vi "KM_fancytorque - ark - V2.vi.vi"() -> ()   [LabVIEW 2016]
uses:
  lorentzian.ctl
  circle corners.ctl
  <vilib>/event_ctls.llb/eventvkey.ctl
  peak -- parameters -- complex fit.ctl
  wavepacket.ctl
  filter method control.ctl
  cursor winow.ctl
  KM_SystemParameters.ctl
  parameters -- scan monitor control.ctl
  plot refs -- filter related.ctl
  cursor window action.ctl
  KM_ControlHFLIcommand.ctl
  KM_file -- read-write control.ctl
  filter - complex - four.vi
  linear interp iiii- complex - z-omega.vi
  peak -- PM find lorenzian - V3.vi
  tale of three indices.vi
  Q -- check range -- i -- real.vi
  filter -- window span logic.vi
  linear interp iiii- complex - z-omega - divide.vi
  linear interpolation iiii- complex.vi
  containing bix.vi
  <vilib>/Analysis/baseanly.llb/A x B.vi
  <vilib>/Analysis/baseanly.llb/Complex A x B.vi
  line -- complex.vi
  Q -- check range -- i -- integer.vi
  peak -- guess at omega -- dzdomega V2.vi
  command stack.vi
  tale of three indices -- check state.vi
  Q - not nan -- real.vi
  Q - not nan -- integer.vi
  peak -- z center from mult phase points.vi
  peak -- estimate for lorentzian.vi
  peak -- fake phase around center.vi
  peak -- get weights.vi
  peak -- four corner circle transformation logic.vi
  peak - fit phase around center - V2.vi
  array - generate range.vi
  circle center from three points.vi
  <vilib>/Utility/error.llb/Clear Errors.vi
  peak -- fit function -- minus arctan.vi
  <vilib>/Analysis/Matrix/Numeric/Conversions/Array To Matrix.vi
  <vilib>/Analysis/Matrix/Numeric/Conversions/Array To Matrix - RA2.vi
  <vilib>/Analysis/baseanly.llb/Inverse Matrix.vi
  <vilib>/Analysis/baseanly.llb/Real Inverse Matrix.vi
  <vilib>/gmath/NumericalOptimization/Nonlinear Curve Fit.vi
  <vilib>/gmath/NumericalOptimization/Nonlinear Curve Fit LM.vi
  KM_filter pipe - plot staff - more - V3.vi
panel:
  in  "Auto-update range":bool
  out "Plot: freq vs T":cluster{i32[], dbl[]}(graph)={[1, 2, 3, 4, 5, 6, 7, 8], [0.0, 0.0, 0.0, 0.0, 0.0, 0.0, 0.0, 0.0]}
  in  "scan monitor control":T1={"gamma acc. frac. - min "=0.3, "gamma acc frac.. - max"=3.0, "peak acc. fraction (af)"=5.0, "min peak acc. window (kHz)"=0.5, "use"=enum."fraction", "abs gamma min(kHz)"=0.005, "abs gamma max(kHz)"=5.0, "# points"=5, "gamma-factor (fa)"=12.0, "interpolate"=enum."line", "init"=TRUE, "Unique strike parameters"=TRUE, "max peak acc. window (kHz)"=10.0, "spacing factor"=1.5, "iterate #"=1, "overwrite ctl?"=FALSE, "write _m files?"=FALSE, "max slope (kHz/sweep)"=0.5, "funnel state"=enum."funnel open"}
  in  "Plot frequency shift":bool=TRUE
  in  "Tab : all plot":enum32{"Page 1"}(tab)
  in  "Save frequency scan":path=path "D:/data/TestFolder/1_test"
  in  "File name":string="lowT_turnonfield"
  in  "ZI HFLI System Parameters IN":T2={"IP Address"="DEV3523", "Start (Hz)"=44300.0, "Stop (Hz)"=44600.0, "Filter Order"=4, "Number of Points"=100, "Precision"=0, "Bandwidth (Hz)"=1.0, "Averaging"=1, "Log Sweep"=FALSE, "Demod"=0} {"Averaging" items=["1"=1, "2"=2, "4"=4, "16"=16, "32"=32, "64"=64]; "Bandwidth (Hz)" format="%#_p"; "Precision" items=["Low", "Med", "High"]; "Number of Points" min=2 max=66000; "Filter Order" items=["6, 1st"=1, "12, 2nd"=2, "18, 3rd"=3, "24, 4th"=4, "30, 5th"=5, "36, 6th"=6, "42, 7th"=7, "48, 8th"=8]; "Stop (Hz)" format="%_5p"; "Start (Hz)" format="%_5p"}
  in  "cursor bracket: All, data window":T3={"left"=43985.294117647056, "right "=45220.58823529412, "center"=44602.94117647059, "window"=1235.294117647063, "cursors"=[0, 1, 2], "relative"=2, "absolute"=2, "fixed vertical offset"=0.0, "vertical offset"=0.0, "skew"=0.0, "default window frac"=0.1, "kind"=enum."symmetric", "skew.left"=0.5, "skew.right"=0.5, "Plot ref"=refnum, "wing order"=enum."forw"}
  in  "Update system parameters":bool
  out "Plot: All":cluster{"all rows":dbl[], "all rows":dbl[]}[](graph)=[{"all rows"=[23781.086279042767, 37884.17530453629, 40730.30165309847, 41954.39033644089, 42636.5910965833, 43072.211915828164, 43374.97472640881, 43597.991322043665, 43769.395219758095, 43905.48114733492, 44016.33986360442, 44108.55436461339, 44186.60243501595, 44253.636077860036, 44311.93853542682, 44363.204457812426, 44408.71822460464, 44449.47114674833, 44486.24066879261, 44519.645208971815, 44550.18295396032, 44578.25983124116, 44604.21002541093, 44628.311259019785, 44650.7963336142, 44671.861957527966, 44691.67557714009, 44710.380719872854, 44728.10121457246, 44744.94455579366, 44761.00460863403, 44776.36380085277, 44791.094912919354, 44805.26255024563, 44818.924362350524, 44832.132059149895, 44844.93226360091, 44857.367231602824, 44869.47546368073, 44881.29222806208, 44892.85001093923, 44904.17890673009, 44915.30695880868, 44926.260459332385, 44937.06421533274, 44947.741787080384, 44958.31570381856, 44968.80766123682, 44979.238704490075, 44989.629400131525, 45000.0, 45010.370599868475, 45020.761295509925, 45031.19233876318, 45041.68429618144, 45052.258212919616, 45062.93578466726, 45073.739540667615, 45084.69304119132, 45095.82109326991, 45107.14998906077, 45118.70777193792, 45130.52453631927, 45142.632768397176, 45155.06773639909, 45167.867940850105, 45181.075637649476, 45194.73744975437, 45208.905087080646, 45223.63619914723, 45238.99539136597, 45255.05544420634, 45271.89878542754, 45289.619280127146, 45308.32442285991, 45328.138042472034, 45349.2036663858, 45371.688740980215, 45395.78997458907, 45421.74016875884, 45449.81704603968, 45480.354791028185, 45513.75933120739, 45550.52885325168, 45591.28177539536, 45636.79554218758, 45688.06146457318, 45746.363922139964, 45813.39756498405, 45891.44563538661, 45983.66013639558, 46094.51885266508, 46230.604780241905, 46402.008677956335, 46625.0252735912, 46927.788084171836, 47363.4089034167, 48045.60966355911, 49269.69834690153, 52115.82469546374], "all rows"=[1.507180397819642e-06, 3.0053428725600797e-06, 3.922075606503711e-06, 2.608239407945581e-06, 2.3153068786215975e-06, 2.1667159786404756e-06, 2.2480663150920602e-06, 2.1591637736680415e-06, 2.0406010131102796e-06, 1.8131660473052188e-06, 2.1641631962096037e-06, 1.6620790138843332e-06, 1.5483188951621796e-06, 1.0039220906155144e-06, 7.603105581707233e-07, -1.1257645296058376e-06, -4.067212706942762e-06, -9.665017348967127e-06, -2.7145929394177068e-05, -0.00015905859596686202, -0.00029765078861135373, -0.0005568586601063002, -7.503199898033523e-05, -2.4381034058832112e-05, -1.3732745859881554e-05, -9.162128154662954e-06, -5.7880575952868944e-06, -4.839254973019342e-06, -2.8674168905364767e-06, -2.511508572255624e-06, -1.9266065464564903e-06, -1.180561993162238e-06, -4.414876509949326e-07, -2.4995144900751636e-07, -2.306090385920931e-06, -3.32898094398004e-07, -2.3974866755640355e-07, 1.019240574116253e-07, 3.263816715050899e-08, 3.291312346419152e-07, 5.720671533295986e-07, 7.264601026105059e-07, 7.144153344906329e-07, 1.1467252526209203e-06, 1.3885442917260242e-07, 1.3569293842464745e-06, 4.986733167554071e-07, 9.04226425622522e-07, 8.405279148001506e-07, 9.635784680639955e-07, 9.025585600632723e-07, 9.53052489210983e-07, 1.064445276409997e-06, 9.414531610527688e-07, 1.1423376391833232e-06, 1.4404747200271967e-06, 1.1572303607929983e-06, 1.1489136925931929e-06, 1.1608344292377982e-06, 1.4063601012768658e-06, 1.1901130130630255e-06, 1.267385218460013e-06, 1.2134881757096428e-06, 1.3140538499450182e-06, 1.4380948660954965e-06, 1.4226762033262723e-06, 1.6676294224025657e-06, 1.4022384399448908e-06, 1.5332878307531674e-06, 1.3371392082792312e-06, 1.4812625899300352e-06, 1.5474023741165714e-06, 1.4765911352317293e-06, 1.5663869417997434e-06, 1.5191387016899292e-06, 1.5814603438757944e-06, 1.527339090381671e-06, 1.3993064074261812e-06, 1.3677070038810398e-06, 1.654406355267649e-06, 1.662451704615306e-06, 1.6023238691482394e-06, 1.643536308331802e-06, 1.715109028918168e-06, 1.7672201376857162e-06, 1.5898175608271295e-06, 1.6967535631888778e-06, 1.744979743776765e-06, 1.8004170427800995e-06, 1.6455601680772773e-06, 1.753509292922102e-06, 1.6387646743650107e-06, 1.8549056202586698e-06, 1.869763756168511e-06, 1.665830966011183e-06, 2.013303355058319e-06, 1.7103469358340893e-06, 1.7213577107899512e-06, 1.7921659681489454e-06, 1.4924510638264252e-06]}, {"all rows"=[23781.086279042767, 37884.17530453629, 40730.30165309847, 41954.39033644089, 42636.5910965833, 43072.211915828164, 43374.97472640881, 43597.991322043665, 43769.395219758095, 43905.48114733492, 44016.33986360442, 44108.55436461339, 44186.60243501595, 44253.636077860036, 44311.93853542682, 44363.204457812426, 44408.71822460464, 44449.47114674833, 44486.24066879261, 44519.645208971815, 44550.18295396032, 44578.25983124116, 44604.21002541093, 44628.311259019785, 44650.7963336142, 44671.861957527966, 44691.67557714009, 44710.380719872854, 44728.10121457246, 44744.94455579366, 44761.00460863403, 44776.36380085277, 44791.094912919354, 44805.26255024563, 44818.924362350524, 44832.132059149895, 44844.93226360091, 44857.367231602824, 44869.47546368073, 44881.29222806208, 44892.85001093923, 44904.17890673009, 44915.30695880868, 44926.260459332385, 44937.06421533274, 44947.741787080384, 44958.31570381856, 44968.80766123682, 44979.238704490075, 44989.629400131525, 45000.0, 45010.370599868475, 45020.761295509925, 45031.19233876318, 45041.68429618144, 45052.258212919616, 45062.93578466726, 45073.739540667615, 45084.69304119132, 45095.82109326991, 45107.14998906077, 45118.70777193792, 45130.52453631927, 45142.632768397176, 45155.06773639909, 45167.867940850105, 45181.075637649476, 45194.73744975437, 45208.905087080646, 45223.63619914723, 45238.99539136597, 45255.05544420634, 45271.89878542754, 45289.619280127146, 45308.32442285991, 45328.138042472034, 45349.2036663858, 45371.688740980215, 45395.78997458907, 45421.74016875884, 45449.81704603968, 45480.354791028185, 45513.75933120739, 45550.52885325168, 45591.28177539536, 45636.79554218758, 45688.06146457318, 45746.363922139964, 45813.39756498405, 45891.44563538661, 45983.66013639558, 46094.51885266508, 46230.604780241905, 46402.008677956335, 46625.0252735912, 46927.788084171836, 47363.4089034167, 48045.60966355911, 49269.69834690153, 52115.82469546374], "all rows"=[0.0007974563535224752, 0.0007996824585144777, 0.000801055863810559, 0.0008023709492684473, 0.0008043035904232198, 0.0008060221240327267, 0.0008079861588657607, 0.0008099138649989499, 0.0008137066342146559, 0.0008166912805273911, 0.0008200120682383414, 0.0008257743088013124, 0.0008309641548394156, 0.0008382418841201335, 0.0008461487511330439, 0.0008631010803868039, 0.0008811271703963326, 0.0009105163414004749, 0.0009569645659724035, 0.0010924084360759998, 0.0012057100706609103, 0.00029661926295813424, 0.0004983682064819104, 0.0006245092460519504, 0.0006642958975118122, 0.000688014953523849, 0.0007036528258253693, 0.0007157261277439108, 0.0007257539872476703, 0.0007312959968075897, 0.0007365652850056019, 0.000741597283698577, 0.0007446082694069566, 0.0007471174935341076, 0.0007503508253399753, 0.000751918924870222, 0.0007545834972275356, 0.0007563965356655345, 0.0007580560809787534, 0.0007597345506328334, 0.0007610640147972753, 0.0007620638516011741, 0.000763219604317757, 0.0007641855095685925, 0.0007646270699688182, 0.0007654766384662939, 0.0007665995562350204, 0.0007680602236370042, 0.0007685370065909853, 0.0007691156724573211, 0.0007697904764320084, 0.0007706588523945321, 0.0007710474382361046, 0.0007717486794004843, 0.0007720769775968043, 0.0007732272174720945, 0.0007736182720170691, 0.0007738807929827457, 0.0007742776555400716, 0.0007749620475055803, 0.0007754371345676591, 0.0007757086490079029, 0.0007762899207278298, 0.0007767543315421529, 0.0007771810290360273, 0.0007776882688728486, 0.0007779256746573937, 0.0007785274443675241, 0.0007789731848669883, 0.0007792025447058807, 0.000779593397699708, 0.000780229163960165, 0.0007805874509397673, 0.0007808925743319777, 0.0007811659957561538, 0.0007818848982870454, 0.0007824298317662446, 0.0007827009109037148, 0.0007832737586205113, 0.0007835664359312226, 0.0007840133213366123, 0.0007843433541846707, 0.0007848029218084065, 0.0007852955640946771, 0.000785941246910104, 0.0007862507459896485, 0.0007870285282892873, 0.000787403374663448, 0.0007878750037518486, 0.0007886287358713888, 0.0007892760304996889, 0.0007898803386809262, 0.0007905251121309694, 0.0007910664952091892, 0.0007919339457060896, 0.0007926132285289055, 0.0007933472670739158, 0.0007941997139364451, 0.0007955754573450963, 0.0007958472103074079]}]
  in  "Tab : everything":T4(tab)
  in  "Tab :  Fit controls":enum32{"complex plane", "complex plane 2"}(tab)
  in  "Plot: fragment - filter":cluster{dbl[], dbl[]}[](graph)=[{[44016.33986360442, 44108.55436461339, 44186.60243501595, 44253.636077860036, 44311.93853542682, 44363.204457812426, 44408.71822460464, 44449.47114674833, 44486.24066879261, 44519.645208971815, 44550.18295396032, 44578.25983124116, 44604.21002541093, 44628.311259019785, 44650.7963336142, 44671.861957527966, 44691.67557714009, 44710.380719872854, 44728.10121457246, 44744.94455579366, 44761.00460863403, 44776.36380085277, 44791.094912919354, 44805.26255024563, 44818.924362350524, 44832.132059149895, 44844.93226360091, 44857.367231602824, 44869.47546368073, 44881.29222806208, 44892.85001093923, 44904.17890673009, 44915.30695880868, 44926.260459332385, 44937.06421533274, 44947.741787080384, 44958.31570381856, 44968.80766123682, 44979.238704490075, 44989.629400131525, 45000.0, 45010.370599868475, 45020.761295509925, 45031.19233876318, 45041.68429618144, 45052.258212919616, 45062.93578466726, 45073.739540667615, 45084.69304119132, 45095.82109326991, 45107.14998906077, 45118.70777193792, 45130.52453631927, 45142.632768397176, 45155.06773639909, 45167.867940850105, 45181.075637649476, 45194.73744975437, 45208.905087080646], [3.2761277517625694e-05, 3.368662392853569e-05, 3.484817959260281e-05, 3.6103896069265395e-05, 3.780540521310197e-05, 4.01312562105535e-05, 4.1697056448412104e-05, 4.347218849800507e-05, 3.7907135227185645e-05, -5.6790609684878474e-05, -0.00016339047566297474, -0.0006374801230611212, -0.0001209044081063004, -4.0885266907126506e-05, -2.0811384583670646e-05, -1.0567441807905433e-05, -3.4639706146223517e-06, 4.146373059885665e-07, 4.783819783945139e-06, 6.487024951166878e-06, 8.345406755318776e-06, 1.0301866106267696e-05, 1.175628931342121e-05, 1.2556906642669138e-05, 1.1355840740066054e-05, 1.3653149534934326e-05, 1.4396450549924569e-05, 1.51720158795756e-05, 1.551153833224406e-05, 1.621032364967834e-05, 1.6771656102487094e-05, 1.716636559117661e-05, 1.7437922034212302e-05, 1.8093758491666083e-05, 1.7224831656009514e-05, 1.8613962643004104e-05, 1.8057064811010596e-05, 1.8808208984914108e-05, 1.886329540863593e-05, 1.9124404198964482e-05, 1.923061546287002e-05, 1.949237776515521e-05, 1.9695602411581522e-05, 1.9748210015891906e-05, 2.0023423103981333e-05, 2.0594351952506144e-05, 2.0415578199513682e-05, 2.0471849694701305e-05, 2.0580663842203036e-05, 2.0986422801630558e-05, 2.0893196741743764e-05, 2.1034651211649477e-05, 2.1124846709259075e-05, 2.133615640300294e-05, 2.1560983405099388e-05, 2.1670341368931204e-05, 2.1966004899596587e-05, 2.1856178916878592e-05, 2.2092467349835007e-05]}, {[44016.33986360442, 44108.55436461339, 44186.60243501595, 44253.636077860036, 44311.93853542682, 44363.204457812426, 44408.71822460464, 44449.47114674833, 44486.24066879261, 44519.645208971815, 44550.18295396032, 44578.25983124116, 44604.21002541093, 44628.311259019785, 44650.7963336142, 44671.861957527966, 44691.67557714009, 44710.380719872854, 44728.10121457246, 44744.94455579366, 44761.00460863403, 44776.36380085277, 44791.094912919354, 44805.26255024563, 44818.924362350524, 44832.132059149895, 44844.93226360091, 44857.367231602824, 44869.47546368073, 44881.29222806208, 44892.85001093923, 44904.17890673009, 44915.30695880868, 44926.260459332385, 44937.06421533274, 44947.741787080384, 44958.31570381856, 44968.80766123682, 44979.238704490075, 44989.629400131525, 45000.0, 45010.370599868475, 45020.761295509925, 45031.19233876318, 45041.68429618144, 45052.258212919616, 45062.93578466726, 45073.739540667615, 45084.69304119132, 45095.82109326991, 45107.14998906077, 45118.70777193792, 45130.52453631927, 45142.632768397176, 45155.06773639909, 45167.867940850105, 45181.075637649476, 45194.73744975437, 45208.905087080646], [4.0456808450971675e-05, 4.6166382765358476e-05, 5.1225852273429576e-05, 5.841507250197021e-05, 6.614053424687782e-05, 8.303814246526989e-05, 0.00010123540346869319, 0.00013110022718033595, 0.00018041604648722388, 0.0003440569052588822, 0.0004878676309891713, -0.00032997943510847485, -0.00025246106113384256, -0.00014257921935351738, -0.00010661530793636916, -8.473961821658563e-05, -7.040545973886184e-05, -5.893282942883901e-05, -4.969397906069325e-05, -4.440818367573857e-05, -3.944291172311682e-05, -3.47471838637017e-05, -3.200913365345908e-05, -2.9623362556086906e-05, -2.598473883380795e-05, -2.4948015024345428e-05, -2.238752166091039e-05, -2.071350043998997e-05, -1.9087580489515707e-05, -1.7532952688762136e-05, -1.6303563123755355e-05, -1.537205078526659e-05, -1.4248588940532444e-05, -1.3418081047746337e-05, -1.2742991914311553e-05, -1.2217836385869973e-05, -1.0918831921894665e-05, -9.602091623528738e-06, -9.124237073053972e-06, -8.593371908314502e-06, -7.924191065159315e-06, -7.094668945941207e-06, -6.7452307505540495e-06, -6.035231686449502e-06, -5.766174006007096e-06, -4.7240714488641515e-06, -4.275528285473716e-06, -4.018974308270025e-06, -3.637134715413381e-06, -3.0337816803440395e-06, -2.520187072239941e-06, -2.275888652409779e-06, -1.6991335260216928e-06, -1.2735291644080309e-06, -8.902410950729081e-07, -3.9469006544365804e-07, -2.2455287754577188e-07, 4.2390483974989707e-07, 8.239377285788486e-07]}, {[44016.33986360442, 44108.55436461339, 44186.60243501595, 44253.636077860036, 44311.93853542682, 44363.204457812426, 44408.71822460464, 44449.47114674833, 44486.24066879261, 44519.645208971815, 44550.18295396032, 44578.25983124116, 44604.21002541093, 44628.311259019785, 44650.7963336142, 44671.861957527966, 44691.67557714009, 44710.380719872854, 44728.10121457246, 44744.94455579366, 44761.00460863403, 44776.36380085277, 44791.094912919354, 44805.26255024563, 44818.924362350524, 44832.132059149895, 44844.93226360091, 44857.367231602824, 44869.47546368073, 44881.29222806208, 44892.85001093923, 44904.17890673009, 44915.30695880868, 44926.260459332385, 44937.06421533274, 44947.741787080384, 44958.31570381856, 44968.80766123682, 44979.238704490075, 44989.629400131525, 45000.0, 45010.370599868475, 45020.761295509925, 45031.19233876318, 45041.68429618144, 45052.258212919616, 45062.93578466726, 45073.739540667615, 45084.69304119132, 45095.82109326991, 45107.14998906077, 45118.70777193792, 45130.52453631927, 45142.632768397176, 45155.06773639909, 45167.867940850105, 45181.075637649476, 45194.73744975437, 45208.905087080646], [0.00014701816589705446, 5.2947847370679395e-05, 3.586999749601753e-05, 3.1697600741825146e-05, 2.8068661982239522e-05, 2.4877700562167582e-05, -2.9345519225219134e-06, -9.646497364317756e-05, -0.00011105523865193785, -0.00011260029387788841, -0.0001102151092777365, -0.00010548502923448127, -9.892636150483591e-05, -9.108805990004969e-05, -8.166768359492782e-05, -6.732857092266447e-05, -4.840812256295664e-05, -8.881774809240911e-06, -5.129018874259853e-06, -2.4353816444433204e-06, -7.710980369969736e-08, 1.873696008523641e-06, 7.12309187311545e-06, 8.810924033841332e-06, 1.0795841782445594e-05, 1.222664583614481e-05, 1.325683629045086e-05, 1.4148715352942893e-05, 1.485097391686723e-05, 1.5453606599141607e-05, 1.59836212952573e-05, 1.6454573479070826e-05, 1.6854885066587522e-05, 1.7212986135172704e-05, 1.7545957318211854e-05, 1.790647313168277e-05, 1.8199235918264806e-05, 1.849666296792747e-05, 1.8745200234560643e-05, 1.8977419600807216e-05, 1.9185250986575222e-05, 1.9394311293179484e-05, 1.9576178823644833e-05, 1.9752084840712014e-05, 1.9904534093105755e-05, 2.009913182683566e-05, 2.0250699742575014e-05, 2.0426693349092594e-05, 2.0588207680667192e-05, 2.0736114275826343e-05, 2.0890732862457536e-05, 2.104847533675035e-05, 2.1209752432146604e-05, 2.137500752540979e-05, 2.154472196296422e-05, 2.171942120615107e-05, 2.189968197026005e-05, 2.2086140572887804e-05, 2.058423683639077e-05]}, {[44016.33986360442, 44108.55436461339, 44186.60243501595, 44253.636077860036, 44311.93853542682, 44363.204457812426, 44408.71822460464, 44449.47114674833, 44486.24066879261, 44519.645208971815, 44550.18295396032, 44578.25983124116, 44604.21002541093, 44628.311259019785, 44650.7963336142, 44671.861957527966, 44691.67557714009, 44710.380719872854, 44728.10121457246, 44744.94455579366, 44761.00460863403, 44776.36380085277, 44791.094912919354, 44805.26255024563, 44818.924362350524, 44832.132059149895, 44844.93226360091, 44857.367231602824, 44869.47546368073, 44881.29222806208, 44892.85001093923, 44904.17890673009, 44915.30695880868, 44926.260459332385, 44937.06421533274, 44947.741787080384, 44958.31570381856, 44968.80766123682, 44979.238704490075, 44989.629400131525, 45000.0, 45010.370599868475, 45020.761295509925, 45031.19233876318, 45041.68429618144, 45052.258212919616, 45062.93578466726, 45073.739540667615, 45084.69304119132, 45095.82109326991, 45107.14998906077, 45118.70777193792, 45130.52453631927, 45142.632768397176, 45155.06773639909, 45167.867940850105, 45181.075637649476, 45194.73744975437, 45208.905087080646], [2.9543349231575067e-05, 6.622263754301442e-06, 5.844751218556552e-05, 8.64760044267736e-05, 0.00011085376326877868, 0.00013228936555530942, 0.0001899199017020701, 0.0001268047312879676, 7.709794022453925e-05, 4.487788907863056e-05, 1.9011848125845024e-05, -2.9428812586780188e-06, -2.2050848559948054e-05, -3.908644422709829e-05, -5.497175404839125e-05, -7.48245432951162e-05, -9.646067867457708e-05, -7.445308489933535e-05, -6.64369863015151e-05, -5.990670073578445e-05, -5.4518222743545405e-05, -4.997964461610519e-05, -4.058641852803419e-05, -3.6480442890336726e-05, -3.189895510595679e-05, -2.839666374119746e-05, -2.558978392515327e-05, -2.326668942343806e-05, -2.127428788444015e-05, -1.9536778585624823e-05, -1.7995476961120325e-05, -1.6629228200940416e-05, -1.5413429638235467e-05, -1.427312636878258e-05, -1.322858621080704e-05, -1.2289689457940276e-05, -1.1401697773020838e-05, -1.055770626391259e-05, -9.768904969492412e-06, -9.045212733640518e-06, -8.373581320203459e-06, -7.72612242758626e-06, -7.097831165359448e-06, -6.513288792999122e-06, -5.938102610698212e-06, -5.376347895838546e-06, -4.824505867648575e-06, -4.3045010686012995e-06, -3.838388250503495e-06, -3.360757028336229e-06, -2.875104779032595e-06, -2.3796404941743624e-06, -1.8730740725888754e-06, -1.3540128814297251e-06, -8.20945026306839e-07, -2.7222004922701913e-07, 2.939734948877061e-07, 8.796342601370182e-07, -3.837799418177113e-06]}]
  in  "scale gauge: Plot: complex plane - filter":dbl(slide)=0.015780000000000002 min=0.0 max=0.3 step=1e-05 scale=0.0001..0.3 scale format="%#_5g"
  in  "Plot: complex plane - filter":cluster{dbl[], dbl[]}[](graph)=[{[2.164163196209603e-06, 1.6620790138843318e-06, 1.5483188951621785e-06, 1.003922090615516e-06, 7.603105581707217e-07, -1.125764529605836e-06, -4.067212706942761e-06, -9.665017348967127e-06, -2.7145929394177068e-05, -0.00015905859596686202, -0.00029765078861135373, -0.0005568586601063002, -7.503199898033523e-05, -2.4381034058832112e-05, -1.3732745859881554e-05, -9.162128154662954e-06, -5.788057595286894e-06, -4.839254973019341e-06, -2.8674168905364776e-06, -2.511508572255625e-06, -1.9266065464564916e-06, -1.180561993162238e-06, -4.41487650994934e-07, -2.499514490075154e-07, -2.3060903859209306e-06, -3.328980943980029e-07, -2.39748667556405e-07, 1.0192405741162429e-07, 3.263816715050799e-08, 3.2913123464191414e-07, 5.720671533295997e-07, 7.264601026105075e-07, 7.144153344906331e-07, 1.146725252620921e-06, 1.38854429172601e-07, 1.3569293842464743e-06, 4.986733167554062e-07, 9.042264256225211e-07, 8.405279148001506e-07, 9.635784680639948e-07, 9.025585600632726e-07, 9.530524892109817e-07, 1.0644452764099977e-06, 9.414531610527702e-07, 1.1423376391833224e-06, 1.4404747200271972e-06, 1.1572303607929979e-06, 1.1489136925931935e-06, 1.1608344292377988e-06, 1.4063601012768644e-06, 1.1901130130630264e-06, 1.267385218460012e-06, 1.2134881757096445e-06, 1.314053849945019e-06, 1.4380948660954975e-06, 1.4226762033262713e-06, 1.6676294224025644e-06, 1.40223843994489e-06, 1.533287830753166e-06], [0.0008200120682383414, 0.0008257743088013124, 0.0008309641548394156, 0.0008382418841201335, 0.0008461487511330439, 0.0008631010803868039, 0.0008811271703963326, 0.0009105163414004749, 0.0009569645659724035, 0.0010924084360759998, 0.0012057100706609103, 0.00029661926295813424, 0.0004983682064819104, 0.0006245092460519504, 0.0006642958975118122, 0.000688014953523849, 0.0007036528258253693, 0.0007157261277439108, 0.0007257539872476703, 0.0007312959968075897, 0.0007365652850056019, 0.000741597283698577, 0.0007446082694069566, 0.0007471174935341076, 0.0007503508253399753, 0.000751918924870222, 0.0007545834972275356, 0.0007563965356655345, 0.0007580560809787534, 0.0007597345506328334, 0.0007610640147972753, 0.0007620638516011741, 0.000763219604317757, 0.0007641855095685925, 0.0007646270699688182, 0.0007654766384662939, 0.0007665995562350204, 0.0007680602236370042, 0.0007685370065909853, 0.0007691156724573211, 0.0007697904764320084, 0.0007706588523945321, 0.0007710474382361046, 0.0007717486794004843, 0.0007720769775968043, 0.0007732272174720945, 0.0007736182720170691, 0.0007738807929827457, 0.0007742776555400716, 0.0007749620475055803, 0.0007754371345676591, 0.0007757086490079029, 0.0007762899207278298, 0.0007767543315421529, 0.0007771810290360273, 0.0007776882688728486, 0.0007779256746573937, 0.0007785274443675241, 0.0007789731848669883]}, {[0.00011561149276827264, 3.002682440455542e-05, 7.692060230687957e-07, -1.0144748546305849e-05, -1.9637151855594426e-05, -2.7983915124523556e-05, -6.907127942448518e-05, -0.00014428237203231066, -0.0001462463645178664, -0.0001398483162704091, -0.00013119701598968923, -0.00012123084716596504, -0.00011018949041649781, -9.841538460038078e-05, -8.538934082025757e-05, -6.662226051630844e-05, -4.297650940535873e-05, -1.0048726402963845e-05, -8.374865021013543e-06, -7.363706425507477e-06, -6.397870381678189e-06, -5.618795156689339e-06, -2.8314162280454252e-06, -2.2012802422878325e-06, -1.3996488958974282e-06, -8.707618370683485e-07, -5.598517179200612e-07, -2.644768396572604e-07, -7.189922546371004e-08, 8.65554524104111e-08, 2.2269002982264067e-07, 3.444623383384534e-07, 4.346181074498293e-07, 5.02351706138215e-07, 5.691898464959058e-07, 6.886221380639299e-07, 7.548424339070842e-07, 8.363676442362791e-07, 8.840190389580596e-07, 9.318060355038263e-07, 9.687069773892912e-07, 1.0127231923770736e-06, 1.0350731315980329e-06, 1.0623646416605325e-06, 1.0692075289902756e-06, 1.1202052303904784e-06, 1.1319144786193212e-06, 1.175106773475547e-06, 1.2174683228111127e-06, 1.243814327775677e-06, 1.2747019852428314e-06, 1.3062136916950533e-06, 1.3384314980301572e-06, 1.3714439761974514e-06, 1.4053472832229624e-06, 1.4402463888279191e-06, 1.4762565015696968e-06, 1.5135047365668567e-06, 1.2134742604624077e-06], [0.0008374316993265817, 0.0007921562586530478, 0.0008382160143834794, 0.0008643673215716006, 0.0008871124002061885, 0.000907112370783746, 0.0009561697716496443, 0.0008720582024550205, 0.0008202915757118585, 0.0007886753793859338, 0.0007641826011931522, 0.000744056516662368, 0.0007271385091583713, 0.0007125432728117717, 0.0006994509566955575, 0.0006837175498817786, 0.0006673778994972156, 0.0006984009144550001, 0.0007070922435772648, 0.0007140835145197028, 0.0007198856091314899, 0.0007247638646116479, 0.0007351571014507161, 0.0007395515003834029, 0.0007444797166907123, 0.0007482258511681108, 0.0007511996032713754, 0.0007536704270221319, 0.0007557741724548584, 0.000757606383367465, 0.0007592305735203202, 0.000760670574610254, 0.0007619474017126729, 0.0007631406913176119, 0.0007642349794941685, 0.0007652335958829972, 0.0007661662556034268, 0.0007670573999000469, 0.0007678830557602971, 0.0007686415890089114, 0.0007693436723094632, 0.0007700226213519139, 0.0007706763232633728, 0.0007712861493741647, 0.0007718811561756034, 0.0007724734701734894, 0.000773045628674837, 0.0007735929066355044, 0.0007740843875991612, 0.0007745837009609922, 0.0007750924356336868, 0.0007756114486952975, 0.0007761420915638375, 0.0007766858230621915, 0.0007772442269431347, 0.0007778190321087946, 0.0007784121360998912, 0.0007790256325639689, 0.0007740839853632468]}, {[0.00017719815539634276, 0.00017630121387286301, 0.00017361392912084328, 0.0001691469066254962, 0.0001629177756838224, 0.0001549511198298295, 0.0001452783798145543, 0.00013393772952378263, 0.00012097392532316176, 0.00010643812942527284, 9.038770797575136e-05, 7.288600465531837e-05, 5.400209069121223e-05, 3.3810492264609395e-05, 1.2390896389835875e-05, -1.0172163573873112e-05, -3.378964153692238e-05, -5.8368330103591184e-05, -8.381122841904143e-05, -0.0001100179249873768, -0.00013688499394994268, -0.00016430640325994027, -0.00019217393314247314, -0.00022037760318855825, -0.0002488061063975551, -0.00027734724845504533, -0.0003058883905125355, -0.00033431689372153236, -0.00036252056376761757, -0.00039038809365015033, -0.0004178095029601479, -0.0004446765719227138, -0.0004708832684910491, -0.0004963261668064994, -0.0005209048553731683, -0.0005445223333362174, -0.0005670853932999264, -0.0005885049891746999, -0.0006086965876013028, -0.000627580501565409, -0.0006450822048858419, -0.0006611326263353634, -0.0006756684222332523, -0.0006886322264338732, -0.0006999728767246449, -0.00070964561673992, -0.000717612272593913, -0.0007238414035355867, -0.0007283084260309338, -0.0007309957107829536, -0.0007318926523064333, -0.0007309957107829536, -0.0007283084260309338, -0.0007238414035355867, -0.000717612272593913, -0.00070964561673992, -0.0006999728767246448, -0.0006886322264338732, -0.0006756684222332522, -0.0006611326263353634, -0.0006450822048858417, -0.0006275805015654089, -0.0006086965876013028, -0.0005885049891746999, -0.0005670853932999264, -0.0005445223333362175, -0.0005209048553731681, -0.0004963261668064994, -0.0004708832684910489, -0.0004446765719227137, -0.0004178095029601479, -0.00039038809365015017, -0.00036252056376761746, -0.00033431689372153203, -0.00030588839051253543, -0.0002773472484550454, -0.0002488061063975549, -0.00022037760318855827, -0.00019217393314247287, -0.00016430640325994017, -0.0001368849939499428, -0.00011001792498737664, -8.381122841904145e-05, -5.836833010359094e-05, -3.37896415369223e-05, -1.0172163573872841e-05, 1.2390896389836037e-05, 3.3810492264609395e-05, 5.4002090691212395e-05, 7.288600465531848e-05, 9.038770797575147e-05, 0.00010643812942527295, 0.00012097392532316176, 0.00013393772952378273, 0.00014527837981455436, 0.0001549511198298296, 0.00016291777568382246, 0.0001691469066254962, 0.00017361392912084328, 0.00017630121387286301], [0.0007511646668095222, 0.0007797058088670124, 0.0008081343120760092, 0.0008363379821220944, 0.0008642055120046272, 0.0008916269213146248, 0.0009184939902771908, 0.0009447006868455261, 0.0009701435851609764, 0.0009947222737276451, 0.0010183397516906945, 0.0010409028116544034, 0.001062322407529177, 0.0010825140059557798, 0.001101397919919886, 0.0011188996232403188, 0.0011349500446898404, 0.0011494858405877292, 0.0011624496447883502, 0.0011737902950791218, 0.001183463035094397, 0.00119142969094839, 0.0011976588218900637, 0.0012021258443854108, 0.0012048131291374305, 0.0012057100706609103, 0.0012048131291374305, 0.0012021258443854106, 0.0011976588218900637, 0.00119142969094839, 0.001183463035094397, 0.0011737902950791218, 0.0011624496447883502, 0.0011494858405877292, 0.0011349500446898404, 0.0011188996232403188, 0.001101397919919886, 0.0010825140059557798, 0.0010623224075291767, 0.0010409028116544032, 0.0010183397516906945, 0.0009947222737276451, 0.0009701435851609763, 0.000944700686845526, 0.0009184939902771906, 0.0008916269213146246, 0.0008642055120046273, 0.0008363379821220944, 0.0008081343120760092, 0.0007797058088670123, 0.0007511646668095221, 0.000722623524752032, 0.0006941950215430351, 0.0006659913514969499, 0.0006381238216144171, 0.0006107024123044195, 0.0005838353433418535, 0.0005576286467735183, 0.000532185748458068, 0.0005076070598913992, 0.0004839895819283499, 0.0004614265219646409, 0.0004400069260898675, 0.0004198153276632647, 0.00040093141369915847, 0.00038342971037872564, 0.000367379288929204, 0.0003528434930313152, 0.00033987968883069416, 0.0003285390385399226, 0.00031886629852464745, 0.0003108996426706545, 0.00030467051172898075, 0.00030020348923363367, 0.00029751620448161394, 0.0002966192629581342, 0.00029751620448161394, 0.00030020348923363367, 0.0003046705117289808, 0.00031089964267065455, 0.0003188662985246474, 0.0003285390385399227, 0.00033987968883069427, 0.00035284349303131525, 0.00036737928892920416, 0.0003834297103787258, 0.00040093141369915863, 0.0004198153276632647, 0.0004400069260898677, 0.0004614265219646411, 0.0004839895819283503, 0.0005076070598913994, 0.000532185748458068, 0.0005576286467735185, 0.0005838353433418538, 0.00061070241230442, 0.0006381238216144173, 0.00066599135149695, 0.0006941950215430355, 0.000722623524752032]}, {[2.0647169757759032e-05, -0.00025766365716535023, 2.1216879120448203e-05], [-3.6446203799929498e-06, -2.1595626027791793e-05, 6.212892029674316e-06]}, {[2.062738720508259e-05, 2.0655096656106253e-05, 2.0682806107129913e-05, 2.0710515558153576e-05, 2.0738225009177235e-05, 2.0765934460200898e-05, 2.0793643911224558e-05, 2.082135336224822e-05, 2.084906281327188e-05, 2.0876772264295543e-05, 2.0904481715319206e-05, 2.0932191166342866e-05, 2.095990061736653e-05, 2.098761006839019e-05, 2.101531951941385e-05, 2.104302897043751e-05, 2.1070738421461174e-05, 2.1098447872484834e-05, 2.1126157323508496e-05, 2.1153866774532156e-05], [-3.130553646146081e-06, -2.672914224135745e-06, -2.215274802125409e-06, -1.7576353801150727e-06, -1.2999959581047367e-06, -8.423565360944006e-07, -3.8471711408406456e-07, 7.29223079262715e-08, 5.305617299366076e-07, 9.882011519469436e-07, 1.4458405739572797e-06, 1.9034799959676157e-06, 2.361119417977952e-06, 2.818758839988288e-06, 3.276398261998624e-06, 3.73403768400896e-06, 4.191677106019296e-06, 4.649316528029632e-06, 5.106955950039968e-06, 5.564595372050304e-06]}, {[-0.00025766365716535023, -0.00025134797605153714, -0.000245032294937724, -0.0002387166138239109, -0.00023240093271009778, -0.00022608525159628466, -0.00021976957048247157, -0.00021345388936865845, -0.00020713820825484533, -0.00020082252714103224, -0.00019450684602721912, -0.000188191164913406, -0.0001818754837995929, -0.0001755598026857798, -0.00016924412157196667, -0.00016292844045815357, -0.00015661275934434046, -0.00015029707823052734, -0.00014398139711671424, -0.00013766571600290112], [-2.1595626027791793e-05, -2.1595626027791793e-05, -2.1595626027791793e-05, -2.1595626027791793e-05, -2.1595626027791793e-05, -2.1595626027791793e-05, -2.1595626027791793e-05, -2.1595626027791793e-05, -2.1595626027791793e-05, -2.1595626027791793e-05, -2.1595626027791793e-05, -2.1595626027791793e-05, -2.1595626027791793e-05, -2.1595626027791793e-05, -2.1595626027791793e-05, -2.1595626027791793e-05, -2.1595626027791793e-05, -2.1595626027791793e-05, -2.1595626027791793e-05, -2.1595626027791793e-05]}]
  out "Plot: dz/domega":cluster{"omega out":dbl[], dbl[]}(graph)={"omega out"=[44016.33986360442, 44108.55436461339, 44186.60243501595, 44253.636077860036, 44311.93853542682, 44363.204457812426, 44408.71822460464, 44449.47114674833, 44486.24066879261, 44519.645208971815, 44550.18295396032, 44578.25983124116, 44604.21002541093, 44628.311259019785, 44650.7963336142, 44671.861957527966, 44691.67557714009, 44710.380719872854, 44728.10121457246, 44744.94455579366, 44761.00460863403, 44776.36380085277, 44791.094912919354, 44805.26255024563, 44818.924362350524, 44832.132059149895, 44844.93226360091, 44857.367231602824, 44869.47546368073, 44881.29222806208, 44892.85001093923, 44904.17890673009, 44915.30695880868, 44926.260459332385, 44937.06421533274, 44947.741787080384, 44958.31570381856, 44968.80766123682, 44979.238704490075, 44989.629400131525, 45000.0, 45010.370599868475, 45020.761295509925, 45031.19233876318, 45041.68429618144, 45052.258212919616, 45062.93578466726, 45073.739540667615, 45084.69304119132, 45095.82109326991, 45107.14998906077, 45118.70777193792, 45130.52453631927, 45142.632768397176, 45155.06773639909, 45167.867940850105, 45181.075637649476, 45194.73744975437, 45208.905087080646], [0.0013387835222186983, 0.0014187431822907154, 0.0009300131865691842, 0.0009300131865691842, 0.0009300131865691842, 0.0009300131865691842, 0.0018027312356804505, 0.0022213527886856383, 0.0024952377217698366, 0.0028082474232261163, 0.0031799375804701015, 0.0035555563844630574, 0.003927973578996738, 0.0042796648789235415, 0.004647505506064143, 0.004499629695175273, 0.005883256814296557, 0.0025782852759954184, 0.0021441635770048507, 0.0018319134257751915, 0.0016010747080372196, 0.001421704604936841, 0.0009249003532260852, 0.0008827202502025644, 0.0006956213430651689, 0.0005743683133790313, 0.0004862829097663184, 0.0004188748716387719, 0.00036774027072074023, 0.0003336228125727867, 0.00030249565593449564, 0.00027622340109327575, 0.00025658723446967964, 0.00023902886779558503, 0.00022124111156535768, 0.00020703184234557566, 0.00019151897007793758, 0.00018145905429931773, 0.00017197552771960266, 0.0001626540643705662, 0.00015465336814599693, 0.00014817741509499208, 0.0001415133952261617, 0.00013480811792346772, 0.0001288227031601723, 0.00012123347331331342, 0.00011383244039375669, 0.00010762633348186863, 0.00010331828200670589, 9.897499239174104e-05, 9.897499239174104e-05, 9.897499239174104e-05, 9.897499239174104e-05, 9.897499239174104e-05, 9.897499239174104e-05, 9.897499239174104e-05, 9.897499239174104e-05, 9.897499239174104e-05, 9.897499239174104e-05]}
  out "Plot: win omega":T5(graph)={"omega out"=[44016.33986360442, 44108.55436461339, 44186.60243501595, 44253.636077860036, 44311.93853542682, 44363.204457812426, 44408.71822460464, 44449.47114674833, 44486.24066879261, 44519.645208971815, 44550.18295396032, 44578.25983124116, 44604.21002541093, 44628.311259019785, 44650.7963336142, 44671.861957527966, 44691.67557714009, 44710.380719872854, 44728.10121457246, 44744.94455579366, 44761.00460863403, 44776.36380085277, 44791.094912919354, 44805.26255024563, 44818.924362350524, 44832.132059149895, 44844.93226360091, 44857.367231602824, 44869.47546368073, 44881.29222806208, 44892.85001093923, 44904.17890673009, 44915.30695880868, 44926.260459332385, 44937.06421533274, 44947.741787080384, 44958.31570381856, 44968.80766123682, 44979.238704490075, 44989.629400131525, 45000.0, 45010.370599868475, 45020.761295509925, 45031.19233876318, 45041.68429618144, 45052.258212919616, 45062.93578466726, 45073.739540667615, 45084.69304119132, 45095.82109326991, 45107.14998906077, 45118.70777193792, 45130.52453631927, 45142.632768397176, 45155.06773639909, 45167.867940850105, 45181.075637649476, 45194.73744975437, 45208.905087080646], "win omega out"=[561.9199676367352, 469.70546662776906, 533.8430903558983, 533.8430903558983, 533.8430903558983, 533.8430903558983, 469.70546662776906, 417.60759039498225, 374.6751811597496, 338.857798187375, 308.6574997155403, 282.9573525354499, 260.9095731245252, 241.8605457798476, 225.2993468218483, 210.82165467370942, 198.10396961161314, 186.88488750842225, 176.9512912258433, 203.82080013011, 229.05597258303897, 252.9809690422917, 299.9688813191606, 286.99569978889485, 275.46412571818655, 265.2022578047763, 256.0662099402907, 247.93498394570634, 240.70644666435692, 234.29414869641187, 228.6247914974956, 223.6361991472295, 219.27568694912043, 215.4987452642963, 212.26797641265875, 209.5522370315448, 207.325949318707, 205.56855306443322, 204.26407698688854, 203.40081312924303, 202.9710823306741, 202.9710823306741, 203.40081312924303, 204.26407698688854, 205.56855306443322, 207.325949318707, 209.5522370315448, 212.26797641265875, 215.4987452642963, 219.27568694912043, 219.27568694912043, 219.27568694912043, 219.27568694912043, 219.27568694912043, 219.27568694912043, 219.27568694912043, 219.27568694912043, 219.27568694912043, 219.27568694912043]}
  out "Plot: phase":cluster{"omega out":dbl[], dbl[]}(graph)={"omega out"=[44016.33986360442, 44108.55436461339, 44186.60243501595, 44253.636077860036, 44311.93853542682, 44363.204457812426, 44408.71822460464, 44449.47114674833, 44486.24066879261, 44519.645208971815, 44550.18295396032, 44578.25983124116, 44604.21002541093, 44628.311259019785, 44650.7963336142, 44671.861957527966, 44691.67557714009, 44710.380719872854, 44728.10121457246, 44744.94455579366, 44761.00460863403, 44776.36380085277, 44791.094912919354, 44805.26255024563, 44818.924362350524, 44832.132059149895, 44844.93226360091, 44857.367231602824, 44869.47546368073, 44881.29222806208, 44892.85001093923, 44904.17890673009, 44915.30695880868, 44926.260459332385, 44937.06421533274, 44947.741787080384, 44958.31570381856, 44968.80766123682, 44979.238704490075, 44989.629400131525, 45000.0, 45010.370599868475, 45020.761295509925, 45031.19233876318, 45041.68429618144, 45052.258212919616, 45062.93578466726, 45073.739540667615, 45084.69304119132, 45095.82109326991, 45107.14998906077, 45118.70777193792, 45130.52453631927, 45142.632768397176, 45155.06773639909, 45167.867940850105, 45181.075637649476, 45194.73744975437, 45208.905087080646], [-3.6946361079029773, -4.034632351867192, -3.168447751835518, -2.792114825303431, -2.591238419743432, -2.4751776508299113, -2.182238680081631, -1.405890268199224, -0.9931515541812361, -0.692932995854262, -0.4317992331175855, -0.2022032678693031, 0.0, 0.179284542566005, 0.3456474631333579, 0.5465352297933839, 0.751038933266539, 1.062755541501061, 1.1046774581940255, 1.140101205492801, 1.17473153972404, 1.2067438312052001, 1.3001460442028527, 1.339226914333243, 1.3889261279059504, 1.4294261461095532, 1.4626921226053744, 1.492568483438804, 1.5186071379668755, 1.5422171432862566, 1.563939661361645, 1.5838990737446146, 1.6019298254033467, 1.6190600772887205, 1.6352470468209521, 1.6510854355846707, 1.6656318257904497, 1.680030698910202, 1.6932850394153292, 1.7057224231540742, 1.7173312223047814, 1.7288229587864175, 1.7398138030367516, 1.7502824181880001, 1.7604051946775252, 1.7711087490340223, 1.7811505813043533, 1.7912212272611159, 1.8003938533133335, 1.80962013231047, 1.819156175416464, 1.8289801029372175, 1.8391230803440388, 1.8496193459471044, 1.860506672127662, 1.8718269018364841, 1.8836265751895178, 1.8959576641696394, 1.8003434827726768]}
  out "Plot: phase around center":cluster{dbl[], dbl[]}[](graph)=[{[44016.33986360442, 44108.55436461339, 44186.60243501595, 44253.636077860036, 44311.93853542682, 44363.204457812426, 44408.71822460464, 44449.47114674833, 44486.24066879261, 44519.645208971815, 44550.18295396032, 44578.25983124116, 44604.21002541093, 44628.311259019785, 44650.7963336142, 44671.861957527966, 44691.67557714009, 44710.380719872854, 44728.10121457246, 44744.94455579366, 44761.00460863403, 44776.36380085277, 44791.094912919354, 44805.26255024563, 44818.924362350524, 44832.132059149895, 44844.93226360091, 44857.367231602824, 44869.47546368073, 44881.29222806208, 44892.85001093923, 44904.17890673009, 44915.30695880868, 44926.260459332385, 44937.06421533274, 44947.741787080384, 44958.31570381856, 44968.80766123682, 44979.238704490075, 44989.629400131525, 45000.0, 45010.370599868475, 45020.761295509925, 45031.19233876318, 45041.68429618144, 45052.258212919616, 45062.93578466726, 45073.739540667615, 45084.69304119132, 45095.82109326991, 45107.14998906077, 45118.70777193792, 45130.52453631927, 45142.632768397176, 45155.06773639909, 45167.867940850105, 45181.075637649476, 45194.73744975437, 45208.905087080646], [-2.5086617505232818, -2.3740100009868046, -2.2093710782522584, -2.006194362241439, -1.7546171948878309, -1.4456704849166695, -1.0766422351223983, -0.659076456813715, -0.2226891216532475, 0.19404475910960567, 0.5617738773107392, 0.8693557735792842, 1.1197289561307298, 1.3219280196455594, 1.4858010669561719, 1.6198596000708083, 1.7308271660800014, 1.8238263608521303, 1.902715605501166, 1.9704031220646774, 2.0290957112678454, 2.0804840836678835, 2.125877640519493, 2.166301820536919, 2.2025685334273994, 2.2353274405298333, 2.265103612006313, 2.2923254486569182, 2.317345595225116, 2.340456763621025, 2.3619038241866863, 2.381893134148053, 2.400599800965017, 2.418173387532456, 2.434742431023349, 2.4504180505595428, 2.465296849229477, 2.4794632652851467, 2.4929914901472965, 2.5059470433079065, 2.5183880736637847, 2.530366441350363, 2.5419286224214144, 2.5531164697683373, 2.5639678567892843, 2.574517224991007, 2.584796052557625, 2.5948332576713624, 2.6046555478118325, 2.6142877242366502, 2.6237529492386247, 2.6330729824935304, 2.642268391789508, 2.6513587426112792, 2.6603627703998116, 2.669298538789299, 2.6781835867147312, 2.6870350669666565, 2.6958698785308943]}, {[44016.33986360442, 44108.55436461339, 44186.60243501595, 44253.636077860036, 44311.93853542682, 44363.204457812426, 44408.71822460464, 44449.47114674833, 44486.24066879261, 44519.645208971815, 44550.18295396032, 44578.25983124116, 44604.21002541093, 44628.311259019785, 44650.7963336142, 44671.861957527966, 44691.67557714009, 44710.380719872854, 44728.10121457246, 44744.94455579366, 44761.00460863403, 44776.36380085277, 44791.094912919354, 44805.26255024563, 44818.924362350524, 44832.132059149895, 44844.93226360091, 44857.367231602824, 44869.47546368073, 44881.29222806208, 44892.85001093923, 44904.17890673009, 44915.30695880868, 44926.260459332385, 44937.06421533274, 44947.741787080384, 44958.31570381856, 44968.80766123682, 44979.238704490075, 44989.629400131525, 45000.0, 45010.370599868475, 45020.761295509925, 45031.19233876318, 45041.68429618144, 45052.258212919616, 45062.93578466726, 45073.739540667615, 45084.69304119132, 45095.82109326991, 45107.14998906077, 45118.70777193792, 45130.52453631927, 45142.632768397176, 45155.06773639909, 45167.867940850105, 45181.075637649476, 45194.73744975437, 45208.905087080646], [-3.6946361079029773, -4.034632351867192, -3.168447751835518, -2.792114825303431, -2.591238419743432, -2.4751776508299113, -2.182238680081631, -1.405890268199224, -0.9931515541812361, -0.692932995854262, -0.4317992331175855, -0.2022032678693031, 0.0, 0.179284542566005, 0.3456474631333579, 0.5465352297933839, 0.751038933266539, 1.062755541501061, 1.1046774581940255, 1.140101205492801, 1.17473153972404, 1.2067438312052001, 1.3001460442028527, 1.339226914333243, 1.3889261279059504, 1.4294261461095532, 1.4626921226053744, 1.492568483438804, 1.5186071379668755, 1.5422171432862566, 1.563939661361645, 1.5838990737446146, 1.6019298254033467, 1.6190600772887205, 1.6352470468209521, 1.6510854355846707, 1.6656318257904497, 1.680030698910202, 1.6932850394153292, 1.7057224231540742, 1.7173312223047814, 1.7288229587864175, 1.7398138030367516, 1.7502824181880001, 1.7604051946775252, 1.7711087490340223, 1.7811505813043533, 1.7912212272611159, 1.8003938533133335, 1.80962013231047, 1.819156175416464, 1.8289801029372175, 1.8391230803440388, 1.8496193459471044, 1.860506672127662, 1.8718269018364841, 1.8836265751895178, 1.8959576641696394, 1.8003434827726768]}]
  out "Plot: fragment":cluster{dbl[], dbl[]}[](graph)=[{[44016.33986360442, 44108.55436461339, 44186.60243501595, 44253.636077860036, 44311.93853542682, 44363.204457812426, 44408.71822460464, 44449.47114674833, 44486.24066879261, 44519.645208971815, 44550.18295396032, 44578.25983124116, 44604.21002541093, 44628.311259019785, 44650.7963336142, 44671.861957527966, 44691.67557714009, 44710.380719872854, 44728.10121457246, 44744.94455579366, 44761.00460863403, 44776.36380085277, 44791.094912919354, 44805.26255024563, 44818.924362350524, 44832.132059149895, 44844.93226360091, 44857.367231602824, 44869.47546368073, 44881.29222806208, 44892.85001093923, 44904.17890673009, 44915.30695880868, 44926.260459332385, 44937.06421533274, 44947.741787080384, 44958.31570381856, 44968.80766123682, 44979.238704490075, 44989.629400131525, 45000.0, 45010.370599868475, 45020.761295509925, 45031.19233876318, 45041.68429618144, 45052.258212919616, 45062.93578466726, 45073.739540667615, 45084.69304119132, 45095.82109326991, 45107.14998906077, 45118.70777193792, 45130.52453631927, 45142.632768397176, 45155.06773639909, 45167.867940850105, 45181.075637649476, 45194.73744975437, 45208.905087080646], [2.184775448590464e-05, 2.134567030357937e-05, 2.1231910184857216e-05, 2.0687513380310553e-05, 2.044390184786576e-05, 1.85578267600892e-05, 1.5616378582752276e-05, 1.001857394072791e-05, -7.462338104482031e-06, -0.00013937500467716698, -0.0002779671973216587, -0.0005371750688166052, -5.534840769064019e-05, -4.697442769137075e-06, 5.950845429813483e-06, 1.0521463135032083e-05, 1.3895533694408143e-05, 1.4844336316675696e-05, 1.681617439915856e-05, 1.7172082717439412e-05, 1.7756984743238545e-05, 1.85030292965328e-05, 1.9242103638700103e-05, 1.943363984068752e-05, 1.7377500903774106e-05, 1.9350693195297034e-05, 1.9443842622138632e-05, 1.978551534710666e-05, 1.9716229456845545e-05, 2.001272252433695e-05, 2.0255658443024637e-05, 2.0410051392305545e-05, 2.039800662418567e-05, 2.0830316542315958e-05, 1.9822445718867638e-05, 2.104052067394151e-05, 2.0182264606450443e-05, 2.0587817715317558e-05, 2.0524119204495188e-05, 2.0647169757759032e-05, 2.058614984975831e-05, 2.063664377890602e-05, 2.0748036566105035e-05, 2.0625044450747807e-05, 2.082592892887836e-05, 2.1124066009722234e-05, 2.0840821650488035e-05, 2.083250498228823e-05, 2.0844425718932836e-05, 2.10899513909719e-05, 2.0873704302758063e-05, 2.095097650815505e-05, 2.089707946540468e-05, 2.0997645139640056e-05, 2.1121686155790535e-05, 2.110626749302131e-05, 2.13512207120976e-05, 2.1085829729639927e-05, 2.1216879120448203e-05]}, {[44016.33986360442, 44108.55436461339, 44186.60243501595, 44253.636077860036, 44311.93853542682, 44363.204457812426, 44408.71822460464, 44449.47114674833, 44486.24066879261, 44519.645208971815, 44550.18295396032, 44578.25983124116, 44604.21002541093, 44628.311259019785, 44650.7963336142, 44671.861957527966, 44691.67557714009, 44710.380719872854, 44728.10121457246, 44744.94455579366, 44761.00460863403, 44776.36380085277, 44791.094912919354, 44805.26255024563, 44818.924362350524, 44832.132059149895, 44844.93226360091, 44857.367231602824, 44869.47546368073, 44881.29222806208, 44892.85001093923, 44904.17890673009, 44915.30695880868, 44926.260459332385, 44937.06421533274, 44947.741787080384, 44958.31570381856, 44968.80766123682, 44979.238704490075, 44989.629400131525, 45000.0, 45010.370599868475, 45020.761295509925, 45031.19233876318, 45041.68429618144, 45052.258212919616, 45062.93578466726, 45073.739540667615, 45084.69304119132, 45095.82109326991, 45107.14998906077, 45118.70777193792, 45130.52453631927, 45142.632768397176, 45155.06773639909, 45167.867940850105, 45181.075637649476, 45194.73744975437, 45208.905087080646], [4.725177540102735e-05, 5.301401596399834e-05, 5.8203862002101587e-05, 6.548159128281952e-05, 7.33884582957299e-05, 9.034078754948988e-05, 0.00010836687755901855, 0.00013775604856316093, 0.0001842042731350895, 0.00031964814323868574, 0.0004329497778235963, -0.00047614102987917977, -0.00027439208635540366, -0.00014825104678536363, -0.00010846439532550178, -8.474533931346502e-05, -6.910746701194474e-05, -5.703416509340322e-05, -4.7006305589643695e-05, -4.146429602972434e-05, -3.61950078317121e-05, -3.1163009138737035e-05, -2.815202343035741e-05, -2.5642799303206396e-05, -2.2409467497338728e-05, -2.0841367967091976e-05, -1.8176795609778427e-05, -1.6363757171779518e-05, -1.4704211858560575e-05, -1.302574220448066e-05, -1.1696278040038751e-05, -1.069644123613989e-05, -9.540688519557063e-06, -8.574783268721492e-06, -8.133222868495806e-06, -7.283654371020116e-06, -6.160736602293655e-06, -4.700069200309822e-06, -4.223286246328754e-06, -3.6446203799929498e-06, -2.969816405305574e-06, -2.101440442781868e-06, -1.7128546012094197e-06, -1.0116134368297423e-06, -6.833152405097149e-07, 4.6692463478048996e-07, 8.579791797551231e-07, 1.120500145431651e-06, 1.5173627027576181e-06, 2.2017546682663158e-06, 2.6768417303451057e-06, 2.948356170588912e-06, 3.529627890515785e-06, 3.994038704838924e-06, 4.420736198713308e-06, 4.927976035534569e-06, 5.165381820079686e-06, 5.767151530210093e-06, 6.212892029674316e-06]}, {[44016.33986360442, 44108.55436461339, 44186.60243501595, 44253.636077860036, 44311.93853542682, 44363.204457812426, 44408.71822460464, 44449.47114674833, 44486.24066879261, 44519.645208971815, 44550.18295396032, 44578.25983124116, 44604.21002541093, 44628.311259019785, 44650.7963336142, 44671.861957527966, 44691.67557714009, 44710.380719872854, 44728.10121457246, 44744.94455579366, 44761.00460863403, 44776.36380085277, 44791.094912919354, 44805.26255024563, 44818.924362350524, 44832.132059149895, 44844.93226360091, 44857.367231602824, 44869.47546368073, 44881.29222806208, 44892.85001093923, 44904.17890673009, 44915.30695880868, 44926.260459332385, 44937.06421533274, 44947.741787080384, 44958.31570381856, 44968.80766123682, 44979.238704490075, 44989.629400131525, 45000.0, 45010.370599868475, 45020.761295509925, 45031.19233876318, 45041.68429618144, 45052.258212919616, 45062.93578466726, 45073.739540667615, 45084.69304119132, 45095.82109326991, 45107.14998906077, 45118.70777193792, 45130.52453631927, 45142.632768397176, 45155.06773639909, 45167.867940850105, 45181.075637649476, 45194.73744975437, 45208.905087080646], [6.870368443368876e-06, -2.761293618358701e-06, -1.5810682025792897e-05, -3.334516207337746e-05, -5.6223533907280176e-05, -8.408644442245929e-05, -0.00011358267720008554, -0.00013732097474452524, -0.0001470252117005101, -0.00014023128640570307, -0.00012205963498879016, -9.986142483312839e-05, -7.859219727522409e-05, -6.028814904457469e-05, -4.526852444011145e-05, -3.316283678297254e-05, -2.3433174132380943e-05, -1.557579804695263e-05, -9.176887644791154e-06, -3.913667755109109e-06, 4.605618928380092e-07, 4.133331284114578e-06, 7.247487699040254e-06, 9.912494331676978e-06, 1.2212902002369498e-05, 1.4214600205586624e-05, 1.5969408652172816e-05, 1.7518455146652288e-05, 1.8894672889761867e-05, 2.0124659333216106e-05, 2.123007059153265e-05, 2.2228676082733063e-05, 2.313516287577644e-05, 2.3961754249607185e-05, 2.471868924726708e-05, 2.5414597392243554e-05, 2.6056793706153545e-05, 2.665151266596461e-05, 2.7204095025363235e-05, 2.7719137982400364e-05, 2.82006166428037e-05, 2.8651982851119082e-05, 2.907624606030288e-05, 2.9476039856472052e-05, 2.9853676957442577e-05, 3.021119489521146e-05, 3.055039412552861e-05, 3.0872869946947154e-05, 3.118003933127676e-05, 3.1473163547967e-05, 3.1753367292244286e-05, 3.2021654890011886e-05, 3.2278924043447545e-05, 3.252597749365153e-05, 3.276353290585433e-05, 3.299223122487879e-05, 3.321264370089385e-05, 3.3425277745718514e-05, 3.363058174620825e-05]}, {[44016.33986360442, 44108.55436461339, 44186.60243501595, 44253.636077860036, 44311.93853542682, 44363.204457812426, 44408.71822460464, 44449.47114674833, 44486.24066879261, 44519.645208971815, 44550.18295396032, 44578.25983124116, 44604.21002541093, 44628.311259019785, 44650.7963336142, 44671.861957527966, 44691.67557714009, 44710.380719872854, 44728.10121457246, 44744.94455579366, 44761.00460863403, 44776.36380085277, 44791.094912919354, 44805.26255024563, 44818.924362350524, 44832.132059149895, 44844.93226360091, 44857.367231602824, 44869.47546368073, 44881.29222806208, 44892.85001093923, 44904.17890673009, 44915.30695880868, 44926.260459332385, 44937.06421533274, 44947.741787080384, 44958.31570381856, 44968.80766123682, 44979.238704490075, 44989.629400131525, 45000.0, 45010.370599868475, 45020.761295509925, 45031.19233876318, 45041.68429618144, 45052.258212919616, 45062.93578466726, 45073.739540667615, 45084.69304119132, 45095.82109326991, 45107.14998906077, 45118.70777193792, 45130.52453631927, 45142.632768397176, 45155.06773639909, 45167.867940850105, 45181.075637649476, 45194.73744975437, 45208.905087080646], [0.00010669394141191656, 0.00011442470683995865, 0.00012201289697327648, 0.00012827070479561541, 0.00013092309311311988, 0.00012628803098546333, 0.00011002715675733092, 8.028898811189729e-05, 4.1752831782931204e-05, 4.389368492957761e-06, -2.3830333142879786e-05, -4.1095533864751884e-05, -4.964166807315919e-05, -5.251631609058823e-05, -5.210680039242151e-05, -4.995112146687379e-05, -4.6954838388705666e-05, -4.362611465050421e-05, -4.024037437521809e-05, -3.694094246490555e-05, -3.37973352969932e-05, -3.083832385239189e-05, -2.8070560531816865e-05, -2.5489055790398844e-05, -2.3083060655913583e-05, -2.083935070735512e-05, -1.874403347105016e-05, -1.678351400176024e-05, -1.4944980572093492e-05, -1.3216618358446075e-05, -1.1587671223150598e-05, -1.0048421182031766e-05, -8.590125833614305e-06, -7.204936895779837e-06, -5.885812937765785e-06, -4.626433480548744e-06, -3.4211181692869437e-06, -2.264752703563409e-06, -1.1527220575827026e-06, -8.085088358165092e-08, 9.546493419257743e-07, 1.957227023785535e-06, 2.930031651432073e-06, 3.875950138784571e-06, 4.797638902994598e-06, 5.697552233305671e-06, 6.5779674457813785e-06, 7.441007264899035e-06, 8.288659821786251e-06, 9.12279661259769e-06, 9.94518871964866e-06, 1.0757521562436922e-05, 1.1561408415384621e-05, 1.2358402903603783e-05, 1.3150010666882926e-05, 1.3937700365000585e-05, 1.472291418407913e-05, 1.550707799373419e-05, 1.6291611298022168e-05]}]
  out "Plot: complex plane":cluster{dbl[], dbl[]}[](graph)=[{[2.164163196209603e-06, 1.6620790138843318e-06, 1.5483188951621785e-06, 1.003922090615516e-06, 7.603105581707217e-07, -1.125764529605836e-06, -4.067212706942761e-06, -9.665017348967127e-06, -2.7145929394177068e-05, -0.00015905859596686202, -0.00029765078861135373, -0.0005568586601063002, -7.503199898033523e-05, -2.4381034058832112e-05, -1.3732745859881554e-05, -9.162128154662954e-06, -5.788057595286894e-06, -4.839254973019341e-06, -2.8674168905364776e-06, -2.511508572255625e-06, -1.9266065464564916e-06, -1.180561993162238e-06, -4.41487650994934e-07, -2.499514490075154e-07, -2.3060903859209306e-06, -3.328980943980029e-07, -2.39748667556405e-07, 1.0192405741162429e-07, 3.263816715050799e-08, 3.2913123464191414e-07, 5.720671533295997e-07, 7.264601026105075e-07, 7.144153344906331e-07, 1.146725252620921e-06, 1.38854429172601e-07, 1.3569293842464743e-06, 4.986733167554062e-07, 9.042264256225211e-07, 8.405279148001506e-07, 9.635784680639948e-07, 9.025585600632726e-07, 9.530524892109817e-07, 1.0644452764099977e-06, 9.414531610527702e-07, 1.1423376391833224e-06, 1.4404747200271972e-06, 1.1572303607929979e-06, 1.1489136925931935e-06, 1.1608344292377988e-06, 1.4063601012768644e-06, 1.1901130130630264e-06, 1.267385218460012e-06, 1.2134881757096445e-06, 1.314053849945019e-06, 1.4380948660954975e-06, 1.4226762033262713e-06, 1.6676294224025644e-06, 1.40223843994489e-06, 1.533287830753166e-06], [0.0008200120682383414, 0.0008257743088013124, 0.0008309641548394156, 0.0008382418841201335, 0.0008461487511330439, 0.0008631010803868039, 0.0008811271703963326, 0.0009105163414004749, 0.0009569645659724035, 0.0010924084360759998, 0.0012057100706609103, 0.00029661926295813424, 0.0004983682064819104, 0.0006245092460519504, 0.0006642958975118122, 0.000688014953523849, 0.0007036528258253693, 0.0007157261277439108, 0.0007257539872476703, 0.0007312959968075897, 0.0007365652850056019, 0.000741597283698577, 0.0007446082694069566, 0.0007471174935341076, 0.0007503508253399753, 0.000751918924870222, 0.0007545834972275356, 0.0007563965356655345, 0.0007580560809787534, 0.0007597345506328334, 0.0007610640147972753, 0.0007620638516011741, 0.000763219604317757, 0.0007641855095685925, 0.0007646270699688182, 0.0007654766384662939, 0.0007665995562350204, 0.0007680602236370042, 0.0007685370065909853, 0.0007691156724573211, 0.0007697904764320084, 0.0007706588523945321, 0.0007710474382361046, 0.0007717486794004843, 0.0007720769775968043, 0.0007732272174720945, 0.0007736182720170691, 0.0007738807929827457, 0.0007742776555400716, 0.0007749620475055803, 0.0007754371345676591, 0.0007757086490079029, 0.0007762899207278298, 0.0007767543315421529, 0.0007771810290360273, 0.0007776882688728486, 0.0007779256746573937, 0.0007785274443675241, 0.0007789731848669883]}, {[1.6835446529981377e-05, 1.611164896228423e-05, 1.3951670979211079e-05, 1.0389576723863285e-05, 5.481542550539662e-06, -6.950289099289815e-07, -8.042729435906129e-06, -1.6445681400793567e-05, -2.5771365232424824e-05, -3.587270932588159e-05, -4.6590409450559584e-05, -5.775544107304894e-05, -6.919172497499637e-05, -8.07189041275633e-05, -9.215518802951075e-05, -0.00010332021965200007, -0.00011403791977667807, -0.00012413926387013486, -0.0001334649477017661, -0.00014186789966665354, -0.00014921560019263066, -0.0001553921716530993, -0.00016030020582642296, -0.00016386230008177074, -0.00016602227806484387, -0.00016674607563254103, -0.00016602227806484387, -0.00016386230008177074, -0.00016030020582642293, -0.0001553921716530993, -0.00014921560019263064, -0.00014186789966665351, -0.0001334649477017661, -0.0001241392638701348, -0.00011403791977667802, -0.00010332021965200007, -9.215518802951073e-05, -8.071890412756329e-05, -6.919172497499633e-05, -5.7755441073048885e-05, -4.659040945055961e-05, -3.587270932588159e-05, -2.5771365232424803e-05, -1.6445681400793533e-05, -8.042729435906088e-06, -6.950289099289544e-07, 5.481542550539662e-06, 1.0389576723863298e-05, 1.3951670979211079e-05, 1.611164896228423e-05], [0.0008118975598312998, 0.0008234019927289428, 0.0008347249938473749, 0.0008456879926949252, 0.0008561180962307902, 0.0008658508154915671, 0.0008747326596804689, 0.0008826235568088801, 0.0008893990627152922, 0.00089495232362407, 0.0008991957612933248, 0.0009020624541761058, 0.000903507192813172, 0.000903507192813172, 0.0009020624541761058, 0.0008991957612933248, 0.00089495232362407, 0.0008893990627152922, 0.0008826235568088801, 0.0008747326596804689, 0.0008658508154915671, 0.0008561180962307902, 0.0008456879926949252, 0.0008347249938473749, 0.0008234019927289428, 0.0008118975598312998, 0.0008003931269336569, 0.0007890701258152248, 0.0007781071269676743, 0.0007676770234318095, 0.0007579443041710325, 0.0007490624599821307, 0.0007411715628537195, 0.0007343960569473074, 0.0007288427960385296, 0.0007245993583692748, 0.0007217326654864938, 0.0007202879268494276, 0.0007202879268494276, 0.0007217326654864938, 0.0007245993583692747, 0.0007288427960385296, 0.0007343960569473074, 0.0007411715628537196, 0.0007490624599821308, 0.0007579443041710326, 0.0007676770234318095, 0.0007781071269676744, 0.0007890701258152249, 0.0008003931269336569]}, {[1.5110167615378753e-05, 6.103619398712895e-06, -2.9029288179529633e-06, -1.1909477034618822e-05, -2.091602525128468e-05, -2.9922573467950538e-05, -3.8929121684616396e-05, -4.7935669901282254e-05, -5.694221811794811e-05, -6.594876633461397e-05, -7.495531455127983e-05, -8.396186276794569e-05, -9.296841098461155e-05, -0.0001019749592012774, -0.00011098150741794326, -0.00011998805563460913, -0.00012899460385127498, -0.00013800115206794082, -0.0001470077002846067, -0.00015601424850127257], [0.000829610626814871, 0.0008278393201165138, 0.0008260680134181568, 0.0008242967067197996, 0.0008225254000214426, 0.0008207540933230854, 0.0008189827866247282, 0.0008172114799263712, 0.000815440173228014, 0.000813668866529657, 0.0008118975598312998, 0.0008101262531329427, 0.0008083549464345856, 0.0008065836397362284, 0.0008048123330378714, 0.0008030410263395142, 0.0008012697196411571, 0.0007994984129428, 0.0007977271062444429, 0.0007959557995460858]}, {[-5.7242247567708675e-05, -5.901355426606579e-05, -6.07848609644229e-05, -6.255616766278002e-05, -6.432747436113713e-05, -6.609878105949425e-05, -6.787008775785137e-05, -6.964139445620848e-05, -7.14127011545656e-05, -7.318400785292271e-05, -7.495531455127983e-05, -7.672662124963694e-05, -7.849792794799406e-05, -8.026923464635118e-05, -8.204054134470828e-05, -8.38118480430654e-05, -8.558315474142253e-05, -8.735446143977963e-05, -8.912576813813674e-05, -9.089707483649388e-05], [0.0007218320776646413, 0.0007308386258813071, 0.000739845174097973, 0.0007488517223146388, 0.0007578582705313046, 0.0007668648187479706, 0.0007758713669646364, 0.0007848779151813023, 0.0007938844633979681, 0.000802891011614634, 0.0008118975598312998, 0.0008209041080479657, 0.0008299106562646315, 0.0008389172044812974, 0.0008479237526979632, 0.000856930300914629, 0.0008659368491312949, 0.0008749433973479607, 0.0008839499455646267, 0.0008929564937812925]}, {[-0.12581156704567317, -0.12708823453845453, -0.1282854883231538, -0.12940258015512787, -0.1304388118883446, -0.13139353591170155, -0.13226615555376173, -0.13305612545565387, -0.13376295191190393, -0.1343861931789849, -0.13492545975139225, -0.1353804146050721, -0.13575077340805036, -0.13603630469813086, -0.1362368300275517, -0.1363522240745094, -0.13638241472148088, -0.13632738310029446, -0.1361871636039221, -0.13596184386498464], [0.053417260283936584, 0.05025634022094903, 0.04706449453126646, 0.04384371801454582, 0.04059602355126935, 0.03732344084475955, 0.03402801515268081, 0.030711806008819943, 0.027376885935944534, 0.02402533915054391, 0.020659260260261342, 0.01728075295483265, 0.013891928691348568, 0.010494905374662722, 0.00709180603377028, 0.003684757494983572, 0.0002758890527351245, -0.0031326688611621164, -0.006538786008965375, -0.009940333678331052]}, {[-0.13964867422565536, -0.14106577514264268, -0.1423947268436589, -0.14363469877715007, -0.14478491600102064, -0.14584465966694687, -0.14681326746963366, -0.14769013406073395, -0.1484747114271715, -0.14916650923363137, -0.14976509512900354, -0.1502700950165882, -0.15068119328789406, -0.1509981330198834, -0.15122071613554053, -0.15134880352766358, -0.15138231514580192, -0.151321230046285, -0.1511655864053117, -0.1509154814950911], [0.05920815528295751, 0.05569953401304133, 0.05215658529749367, 0.04858152336393376, 0.04497658250969688, 0.041344015705471006, 0.0376860931872636, 0.034005101037578034, 0.03030333975668633, 0.02658312282489164, 0.022846775256677988, 0.01909663214765214, 0.015335037215184807, 0.011564341333663518, 0.007786901065272907, 0.004005077187219661, 0.00022123321632388354, -0.003562266068102054, -0.0073430561021636705, -0.011118774015159573]}, {[0.00011561149276827264, 3.002682440455542e-05, 7.692060230687957e-07, -1.0144748546305849e-05, -1.9637151855594426e-05, -2.7983915124523556e-05, -6.907127942448518e-05, -0.00014428237203231066, -0.0001462463645178664, -0.0001398483162704091, -0.00013119701598968923, -0.00012123084716596504, -0.00011018949041649781, -9.841538460038078e-05, -8.538934082025757e-05, -6.662226051630844e-05, -4.297650940535873e-05, -1.0048726402963845e-05, -8.374865021013543e-06, -7.363706425507477e-06, -6.397870381678189e-06, -5.618795156689339e-06, -2.8314162280454252e-06, -2.2012802422878325e-06, -1.3996488958974282e-06, -8.707618370683485e-07, -5.598517179200612e-07, -2.644768396572604e-07, -7.189922546371004e-08, 8.65554524104111e-08, 2.2269002982264067e-07, 3.444623383384534e-07, 4.346181074498293e-07, 5.02351706138215e-07, 5.691898464959058e-07, 6.886221380639299e-07, 7.548424339070842e-07, 8.363676442362791e-07, 8.840190389580596e-07, 9.318060355038263e-07, 9.687069773892912e-07, 1.0127231923770736e-06, 1.0350731315980329e-06, 1.0623646416605325e-06, 1.0692075289902756e-06, 1.1202052303904784e-06, 1.1319144786193212e-06, 1.175106773475547e-06, 1.2174683228111127e-06, 1.243814327775677e-06, 1.2747019852428314e-06, 1.3062136916950533e-06, 1.3384314980301572e-06, 1.3714439761974514e-06, 1.4053472832229624e-06, 1.4402463888279191e-06, 1.4762565015696968e-06, 1.5135047365668567e-06, 1.2134742604624077e-06], [0.0008374316993265817, 0.0007921562586530478, 0.0008382160143834794, 0.0008643673215716006, 0.0008871124002061885, 0.000907112370783746, 0.0009561697716496443, 0.0008720582024550205, 0.0008202915757118585, 0.0007886753793859338, 0.0007641826011931522, 0.000744056516662368, 0.0007271385091583713, 0.0007125432728117717, 0.0006994509566955575, 0.0006837175498817786, 0.0006673778994972156, 0.0006984009144550001, 0.0007070922435772648, 0.0007140835145197028, 0.0007198856091314899, 0.0007247638646116479, 0.0007351571014507161, 0.0007395515003834029, 0.0007444797166907123, 0.0007482258511681108, 0.0007511996032713754, 0.0007536704270221319, 0.0007557741724548584, 0.000757606383367465, 0.0007592305735203202, 0.000760670574610254, 0.0007619474017126729, 0.0007631406913176119, 0.0007642349794941685, 0.0007652335958829972, 0.0007661662556034268, 0.0007670573999000469, 0.0007678830557602971, 0.0007686415890089114, 0.0007693436723094632, 0.0007700226213519139, 0.0007706763232633728, 0.0007712861493741647, 0.0007718811561756034, 0.0007724734701734894, 0.000773045628674837, 0.0007735929066355044, 0.0007740843875991612, 0.0007745837009609922, 0.0007750924356336868, 0.0007756114486952975, 0.0007761420915638375, 0.0007766858230621915, 0.0007772442269431347, 0.0007778190321087946, 0.0007784121360998912, 0.0007790256325639689, 0.0007740839853632468]}]
  in  "scale gauge: Plot: complex plane":dbl(slide)=0.013730000000000001 min=0.0 max=0.3 step=1e-05 scale=0.0001..1.0 scale format="%#_2g"
  out "window width (kHz)":dbl=76.27809365793496
  out "window center (kHz)":dbl=3399.029286744401
  out "# of points in window":dbl=953.475933538175
  in  "use fast fit?":bool
  out "pm lorentzian":T6={"Amplitude"=0.029322961991943352, "omega(0)"=44504.09928588319, "Gamma"=319.4543943914367, "phase"=-1.37660592159058, "Q"=139.31284110417033, "Norm  Ampl"=nan, "z (inf)"=1.5110167615378767e-05+0.000829610626814871i, "4corners"={"z (-pi/2)"=-5.7242247567708675e-05+0.0007218320776646413i, "z(inf)"=1.5110167615378767e-05+0.000829610626814871i, "z (pi/2)"=-9.266838153485098e-05+0.0009019630419979584i, "z center"=-7.495531455127983e-05+0.0008118975598312998i, "z(0)"=-0.0001650207967179384+0.0007941844928477286i, "radius"=9.17907610812612e-05}} {"z (inf)" format="%#9_9f"; "Q" format="%#9_9f"; "phase" format="%#9_9f"; "Gamma" format="%#9_9f"; "omega(0)" format="%#9_9f"}
  in  "plot staff":enum16{"plot", "do not plot", "a"}(ring)
  in  "Take data":bool
  in  "Tab : parameters":enum32{"Page 1"}(tab)
  out "VKey":T8
  out "Char":i16=101
  out "Voltage out":cdb[](array[numeric])=[1.507180397819642e-06+0.0007974563535224752i, 3.0053428725600797e-06+0.0007996824585144777i, 3.922075606503711e-06+0.000801055863810559i, 2.608239407945581e-06+0.0008023709492684473i, 2.3153068786215975e-06+0.0008043035904232198i, 2.1667159786404756e-06+0.0008060221240327267i, 2.2480663150920602e-06+0.0008079861588657607i, 2.1591637736680415e-06+0.0008099138649989499i, 2.0406010131102796e-06+0.0008137066342146559i, 1.8131660473052188e-06+0.0008166912805273911i, 2.1641631962096037e-06+0.0008200120682383414i, 1.6620790138843332e-06+0.0008257743088013124i, 1.5483188951621796e-06+0.0008309641548394156i, 1.0039220906155144e-06+0.0008382418841201335i, 7.603105581707233e-07+0.0008461487511330439i, -1.1257645296058376e-06+0.0008631010803868039i, -4.067212706942762e-06+0.0008811271703963326i, -9.665017348967127e-06+0.0009105163414004749i, -2.7145929394177068e-05+0.0009569645659724035i, -0.00015905859596686202+0.0010924084360759998i, -0.00029765078861135373+0.0012057100706609103i, -0.0005568586601063002+0.00029661926295813424i, -7.503199898033523e-05+0.0004983682064819104i, -2.4381034058832112e-05+0.0006245092460519504i, -1.3732745859881554e-05+0.0006642958975118122i, -9.162128154662954e-06+0.000688014953523849i, -5.7880575952868944e-06+0.0007036528258253693i, -4.839254973019342e-06+0.0007157261277439108i, -2.8674168905364767e-06+0.0007257539872476703i, -2.511508572255624e-06+0.0007312959968075897i, -1.9266065464564903e-06+0.0007365652850056019i, -1.180561993162238e-06+0.000741597283698577i, -4.414876509949326e-07+0.0007446082694069566i, -2.4995144900751636e-07+0.0007471174935341076i, -2.306090385920931e-06+0.0007503508253399753i, -3.32898094398004e-07+0.000751918924870222i, -2.3974866755640355e-07+0.0007545834972275356i, 1.019240574116253e-07+0.0007563965356655345i, 3.263816715050899e-08+0.0007580560809787534i, 3.291312346419152e-07+0.0007597345506328334i, 5.720671533295986e-07+0.0007610640147972753i, 7.264601026105059e-07+0.0007620638516011741i, 7.144153344906329e-07+0.000763219604317757i, 1.1467252526209203e-06+0.0007641855095685925i, 1.3885442917260242e-07+0.0007646270699688182i, 1.3569293842464745e-06+0.0007654766384662939i, 4.986733167554071e-07+0.0007665995562350204i, 9.04226425622522e-07+0.0007680602236370042i, 8.405279148001506e-07+0.0007685370065909853i, 9.635784680639955e-07+0.0007691156724573211i, 9.025585600632723e-07+0.0007697904764320084i, 9.53052489210983e-07+0.0007706588523945321i, 1.064445276409997e-06+0.0007710474382361046i, 9.414531610527688e-07+0.0007717486794004843i, 1.1423376391833232e-06+0.0007720769775968043i, 1.4404747200271967e-06+0.0007732272174720945i, 1.1572303607929983e-06+0.0007736182720170691i, 1.1489136925931929e-06+0.0007738807929827457i, 1.1608344292377982e-06+0.0007742776555400716i, 1.4063601012768658e-06+0.0007749620475055803i, 1.1901130130630255e-06+0.0007754371345676591i, 1.267385218460013e-06+0.0007757086490079029i, 1.2134881757096428e-06+0.0007762899207278298i, 1.3140538499450182e-06+0.0007767543315421529i, 1.4380948660954965e-06+0.0007771810290360273i, 1.4226762033262723e-06+0.0007776882688728486i, 1.6676294224025657e-06+0.0007779256746573937i, 1.4022384399448908e-06+0.0007785274443675241i, 1.5332878307531674e-06+0.0007789731848669883i, 1.3371392082792312e-06+0.0007792025447058807i, 1.4812625899300352e-06+0.000779593397699708i, 1.5474023741165714e-06+0.000780229163960165i, 1.4765911352317293e-06+0.0007805874509397673i, 1.5663869417997434e-06+0.0007808925743319777i, 1.5191387016899292e-06+0.0007811659957561538i, 1.5814603438757944e-06+0.0007818848982870454i, 1.527339090381671e-06+0.0007824298317662446i, 1.3993064074261812e-06+0.0007827009109037148i, 1.3677070038810398e-06+0.0007832737586205113i, 1.654406355267649e-06+0.0007835664359312226i, 1.662451704615306e-06+0.0007840133213366123i, 1.6023238691482394e-06+0.0007843433541846707i, 1.643536308331802e-06+0.0007848029218084065i, 1.715109028918168e-06+0.0007852955640946771i, 1.7672201376857162e-06+0.000785941246910104i, 1.5898175608271295e-06+0.0007862507459896485i, 1.6967535631888778e-06+0.0007870285282892873i, 1.744979743776765e-06+0.000787403374663448i, 1.8004170427800995e-06+0.0007878750037518486i, 1.6455601680772773e-06+0.0007886287358713888i, 1.753509292922102e-06+0.0007892760304996889i, 1.6387646743650107e-06+0.0007898803386809262i, 1.8549056202586698e-06+0.0007905251121309694i, 1.869763756168511e-06+0.0007910664952091892i, 1.665830966011183e-06+0.0007919339457060896i, 2.013303355058319e-06+0.0007926132285289055i, 1.7103469358340893e-06+0.0007933472670739158i, 1.7213577107899512e-06+0.0007941997139364451i, 1.7921659681489454e-06+0.0007955754573450963i, 1.4924510638264252e-06+0.0007958472103074079i]
  out "Freq out":dbl[](array[numeric])=[23781.086279042767, 37884.17530453629, 40730.30165309847, 41954.39033644089, 42636.5910965833, 43072.211915828164, 43374.97472640881, 43597.991322043665, 43769.395219758095, 43905.48114733492, 44016.33986360442, 44108.55436461339, 44186.60243501595, 44253.636077860036, 44311.93853542682, 44363.204457812426, 44408.71822460464, 44449.47114674833, 44486.24066879261, 44519.645208971815, 44550.18295396032, 44578.25983124116, 44604.21002541093, 44628.311259019785, 44650.7963336142, 44671.861957527966, 44691.67557714009, 44710.380719872854, 44728.10121457246, 44744.94455579366, 44761.00460863403, 44776.36380085277, 44791.094912919354, 44805.26255024563, 44818.924362350524, 44832.132059149895, 44844.93226360091, 44857.367231602824, 44869.47546368073, 44881.29222806208, 44892.85001093923, 44904.17890673009, 44915.30695880868, 44926.260459332385, 44937.06421533274, 44947.741787080384, 44958.31570381856, 44968.80766123682, 44979.238704490075, 44989.629400131525, 45000.0, 45010.370599868475, 45020.761295509925, 45031.19233876318, 45041.68429618144, 45052.258212919616, 45062.93578466726, 45073.739540667615, 45084.69304119132, 45095.82109326991, 45107.14998906077, 45118.70777193792, 45130.52453631927, 45142.632768397176, 45155.06773639909, 45167.867940850105, 45181.075637649476, 45194.73744975437, 45208.905087080646, 45223.63619914723, 45238.99539136597, 45255.05544420634, 45271.89878542754, 45289.619280127146, 45308.32442285991, 45328.138042472034, 45349.2036663858, 45371.688740980215, 45395.78997458907, 45421.74016875884, 45449.81704603968, 45480.354791028185, 45513.75933120739, 45550.52885325168, 45591.28177539536, 45636.79554218758, 45688.06146457318, 45746.363922139964, 45813.39756498405, 45891.44563538661, 45983.66013639558, 46094.51885266508, 46230.604780241905, 46402.008677956335, 46625.0252735912, 46927.788084171836, 47363.4089034167, 48045.60966355911, 49269.69834690153, 52115.82469546374]
  in  "parameters: complex fit":T9={"main VI path"=path "", "scale factor"=3.0, "# of grid points"=200, "parameters: wavepacket"={"R"=0.5, "wave number"=22.0, "delta k"=7.0, "radii vector"=[], "radial section"=[], "wave vector"=22.0, "wavepacket is"=TRUE}, "span"=0.27789, "interference ?"=enum."cp z center", "filter method"=enum."three"} {"span" min=0.0 max=0.5 step=1e-05 scale=0.0001..0.5 scale format="%#_5f"; "parameters: wavepacket"."delta k" format="%#_3f"; "parameters: wavepacket"."wave number" format="%#_3f"; "parameters: wavepacket"."R" format="%#_3f"}
  # "three strikes"
  # "search window"
  # "linear extrapolation"
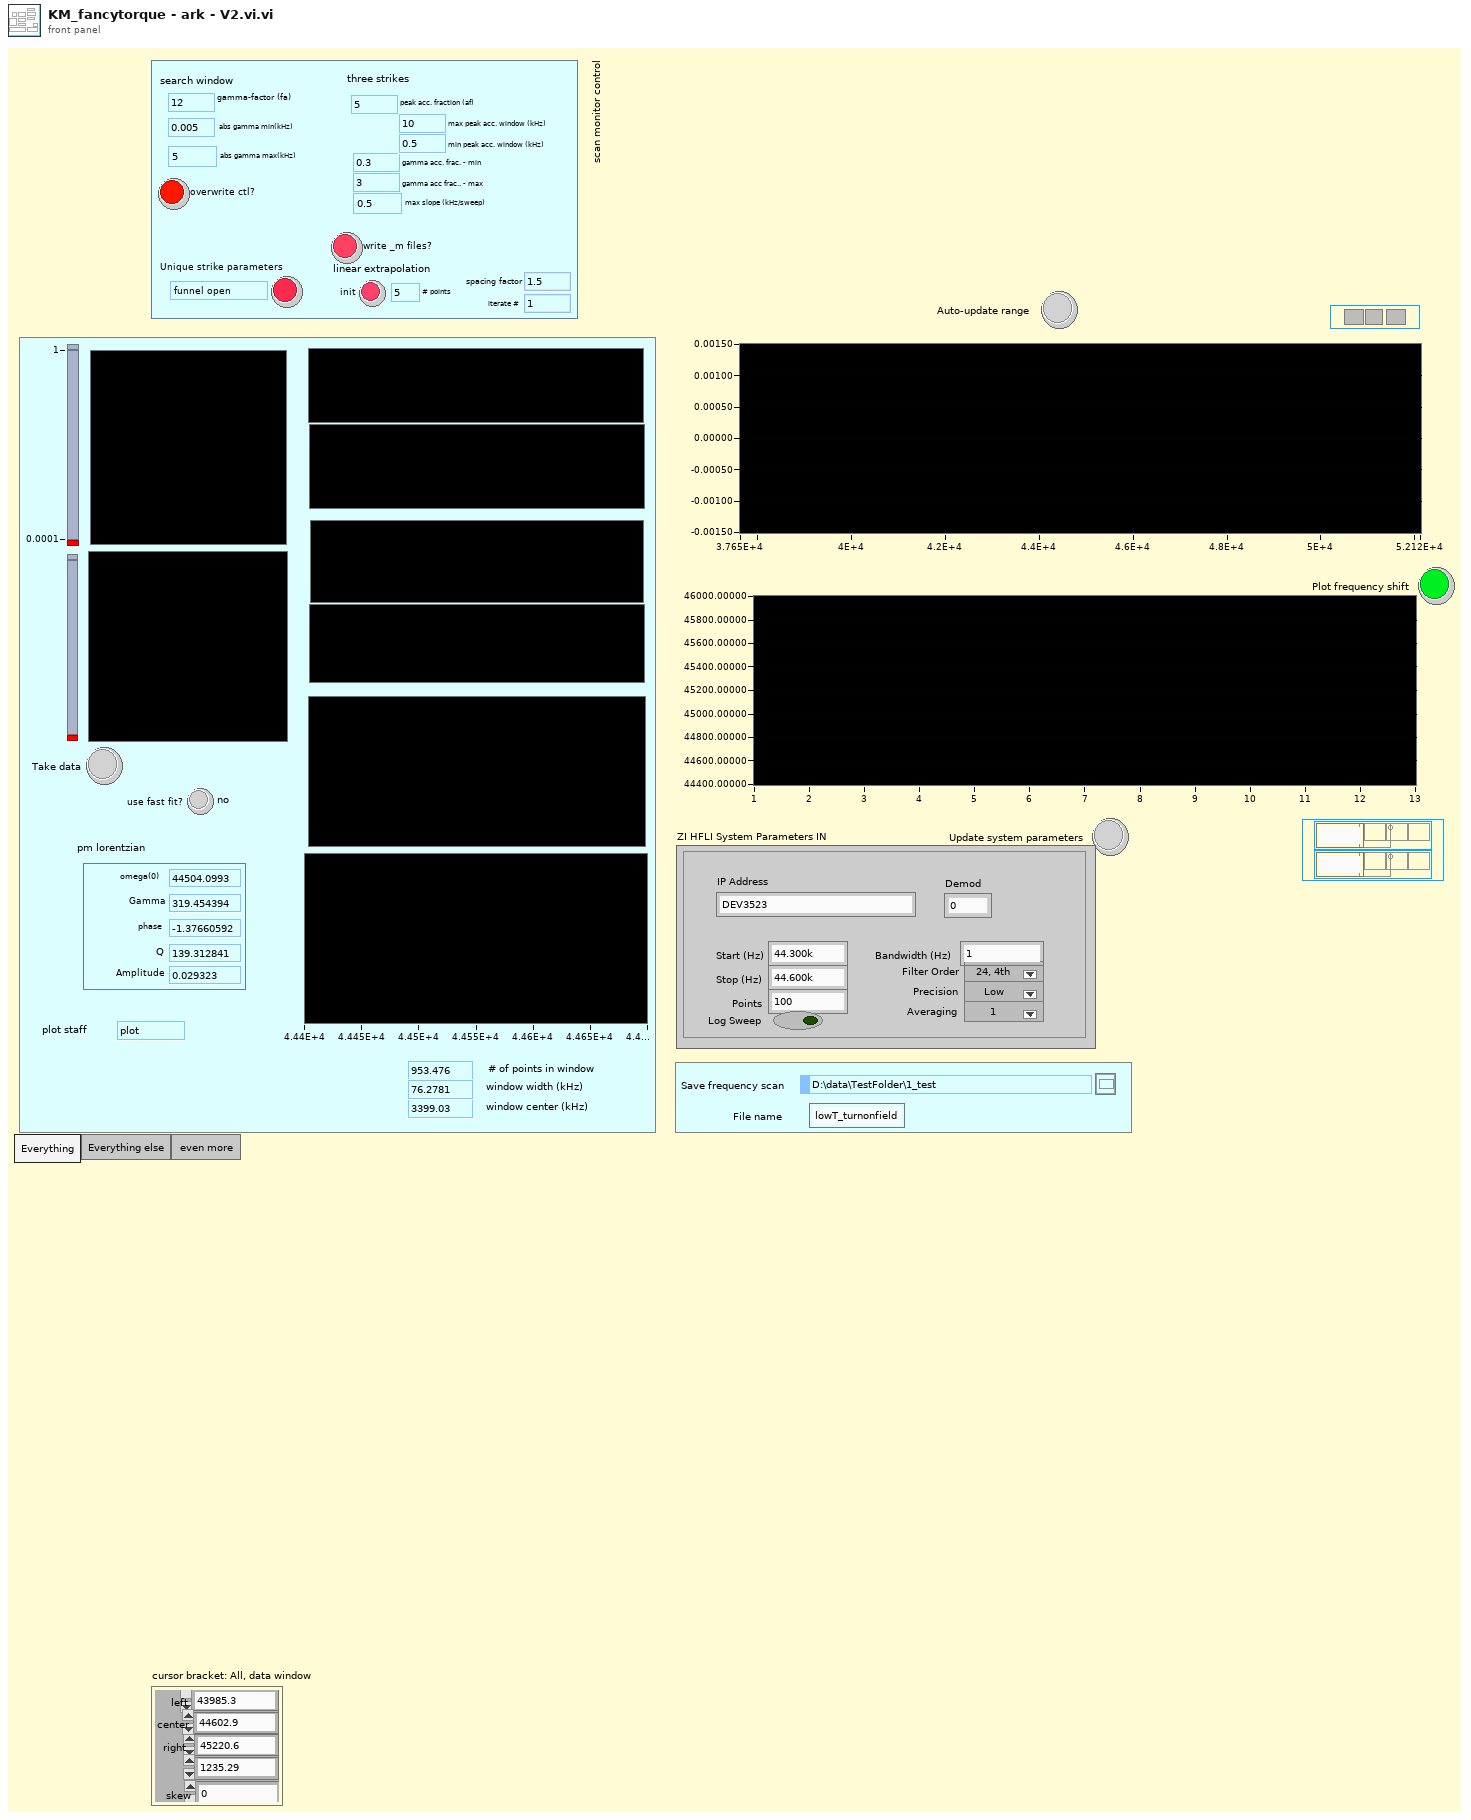
[diagram p1: front panel]
types:
  T1 = typedef "parameters -- scan monitor control.ctl" = cluster{"gamma acc. frac. - min ":dbl, "gamma acc frac.. - max":dbl, "peak acc. fraction (af)":dbl, "min peak acc. window (kHz)":dbl, "use":enum16{"window", "fraction"}, "abs gamma min(kHz)":dbl, "abs gamma max(kHz)":dbl, "# points":i32, "gamma-factor (fa)":dbl, "interpolate":enum16{"line", "last"}, "init":bool, "Unique strike parameters":bool, "max peak acc. window (kHz)":dbl, "spacing factor":dbl, "iterate #":i32, "overwrite ctl?":bool, "write _m files?":bool, "max slope (kHz/sweep)":dbl, "funnel state":enum16{"funnel open", "funnel closed"}}
  T2 = typedef "KM_SystemParameters.ctl" = cluster{"IP Address":string, "Start (Hz)":dbl, "Stop (Hz)":dbl, "Filter Order":i32, "Number of Points":i32, "Precision":u16, "Bandwidth (Hz)":dbl, "Averaging":u16, "Log Sweep":bool, "Demod":i32}
  T3 = typedef "cursor winow.ctl" = cluster{"left":dbl, "right ":dbl, "center":dbl, "window":dbl, "cursors":i32[], "relative":i32, "absolute":i32, "fixed vertical offset":dbl, "vertical offset":dbl, "skew":dbl, "default window frac":dbl, "kind":enum16{"symmetric", "skewed", "fancy"}, "skew.left":dbl, "skew.right":dbl, "Plot ref":refnum<vi>, "wing order":enum16{"forw", "back"}}
  T4 = enum32{"Everything", "Everything else", "even more "}
  T5 = cluster{"omega out":dbl[], "win omega out":dbl[]}
  T6 = typedef "lorentzian.ctl" = cluster{"Amplitude":dbl, "omega(0)":dbl, "Gamma":dbl, "phase":dbl, "Q":dbl, "Norm  Ampl":dbl, "z (inf)":cdb, "4corners":T7}
  T7 = typedef "circle corners.ctl" = cluster{"z (-pi/2)":cdb, "z(inf)":cdb, "z (pi/2)":cdb, "z center":cdb, "z(0)":cdb, "radius":dbl}
  T8 = typedef "eventvkey.ctl" = enum16{"ASCII", "Enter", "Return", "Shift", "Ctrl", "Alt", "Cmd", "Opt", "Caps", "NumLock", "Clear", "Break", "Up", "Down", "Left", "Right", "Insert", "Delete", "Home", "End", "PageUp", "PageDown", "Escape", "Help", "Pause", "ScrollLock", "F1", "F2", "F3", "F4", "F5", "F6", "F7", "F8", "F9", "F10", "F11", "F12", "F13", "F14", "F15", "F16", "F17", "F18", "F19", "F20", "F21", "F22", "F23", "F24", "Play", "VolumeUp", "VolumeDown", "Mute", "Two Byte Char"}
  T9 = typedef "peak -- parameters -- complex fit.ctl" = cluster{"main VI path":path, "scale factor":dbl, "# of grid points":i32, "parameters: wavepacket":T10, "span":dbl, "interference ?":enum16{"cp z center", "pm zcenter", "fancy"}, "filter method":T11}
  T10 = typedef "wavepacket.ctl" = cluster{"R":dbl, "wave number":dbl, "delta k":dbl, "radii vector":dbl[], "radial section":cdb[], "wave vector":dbl, "wavepacket is":bool}
  T11 = typedef "filter method control.ctl" = enum16{"four", "five", "one", "two", "three", "zero", "minus one", "minus two"}
  T12 = typedef "cursor window action.ctl" = enum16{"balance", "h. offset change", "cursor moves", "change center", "change window", "init", "check", "reset", "set y to middle", "idle", "-write all Y", "-write left.X", "-write center.X", "-write right.X", "-write all X", "-change center", "-change window", "-change skew", "-read cursor 2", "-read cursor 1", "-read cursor 0", "-read all cursors", "-reset", "-read plot scale", "-set y to middle", "-Q: center.Y is visible", "-Q: window is visible", "-parse center.Y", "-right left from center", "-left move", "-right move", "-set center.Y", "-empty", "-set cursors to default", "-check", "-write center.Y", "-copy cursor 1", "-copy cursor 0", "-copy cursor 2", "move right", "move left", "shrink", "broaden", "skew up", "skew down", "-write plot scale", "zoom X", "change cen&win", "zoom to all data"}
  T13 = typedef "plot refs -- filter related.ctl" = cluster{"Plot: complex plane - filter":refnum<vi>, "Plot: dz/domega":refnum<vi>, "Plot: fragment filter":refnum<vi>, "Plot: win omega":refnum<vi>, "Plot: phase":refnum<vi>, "Plot: phase around center":refnum<vi>, "Plot: complex plane":refnum<vi>, "Plot: fragment":refnum<vi>}
  T14 = typedef "KM_ControlHFLIcommand.ctl" = enum16{"Initialize", "Scan frequency"}
  T15 = typedef "KM_file -- read-write control.ctl" = enum16{"read", "write all", "append one line"}
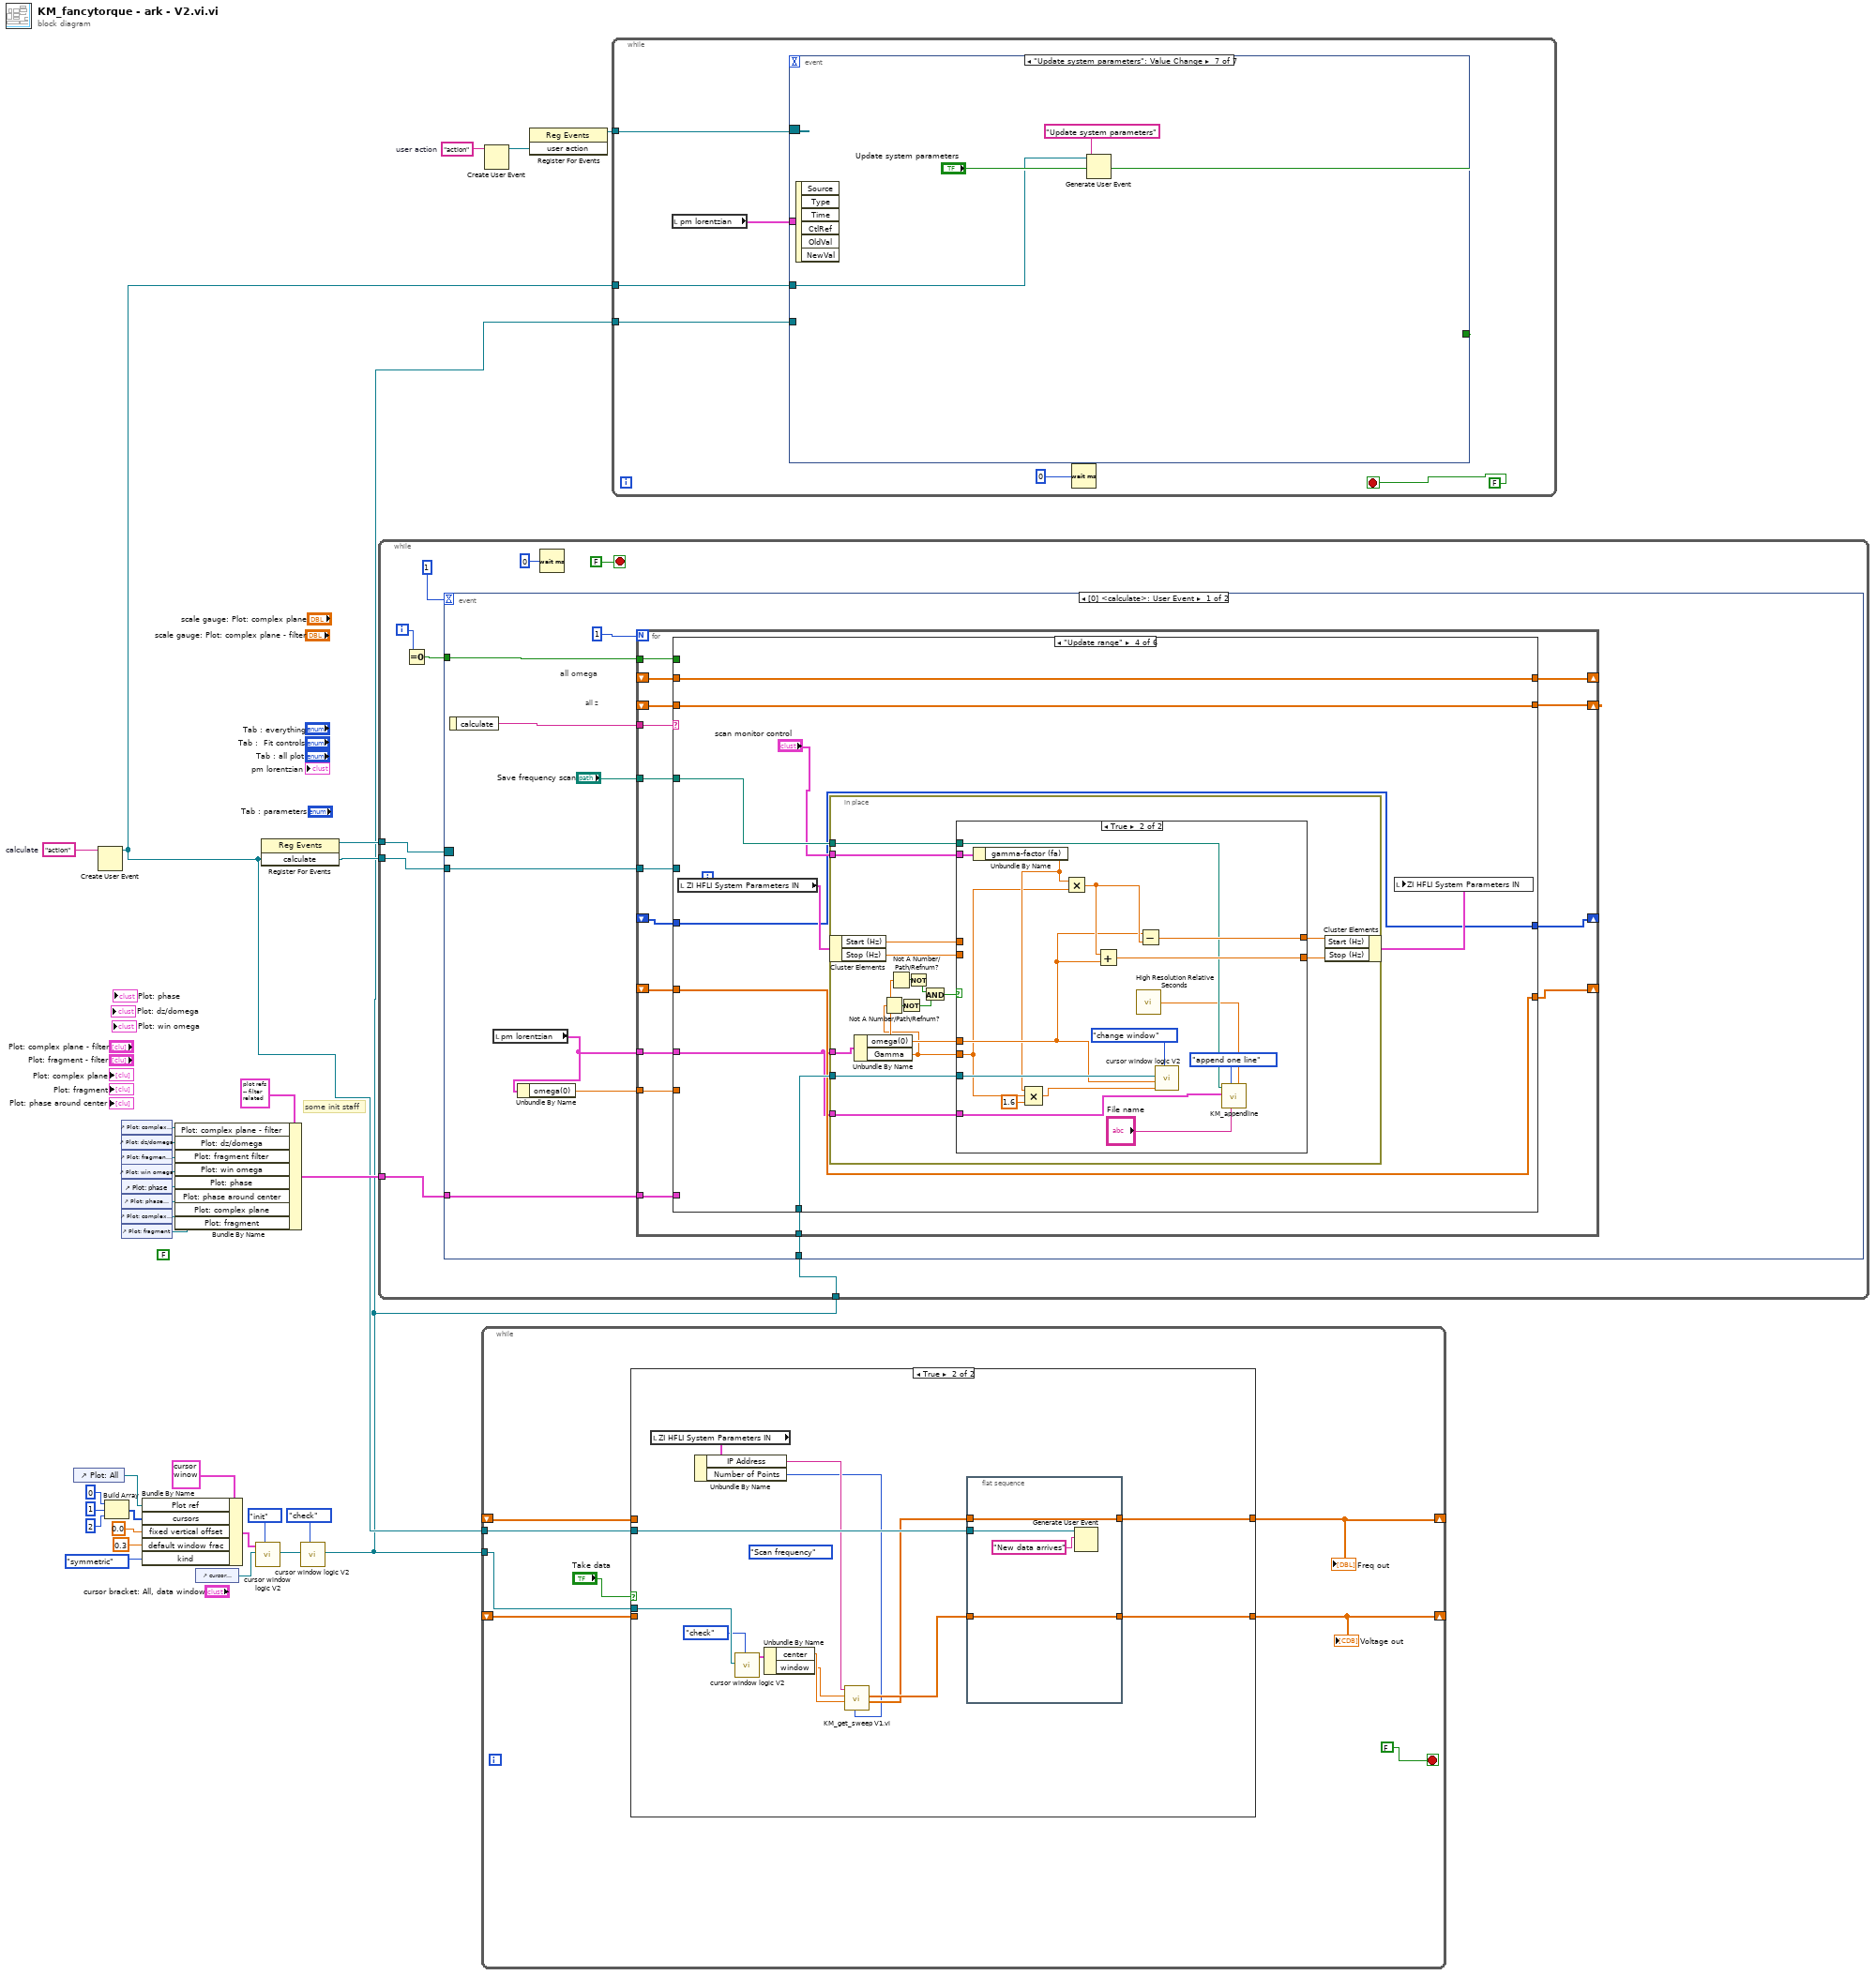
[diagram p0: block diagram]
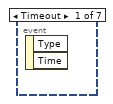
[diagram p3: hidden frame]
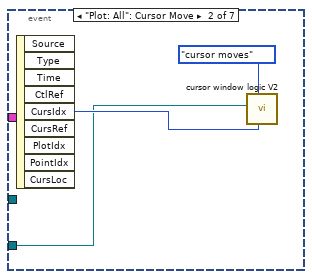
[diagram p4: hidden frame]
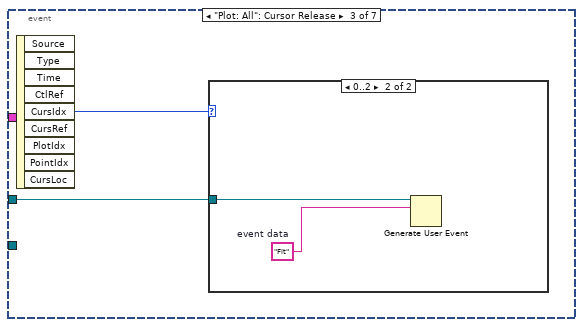
[diagram p5: hidden frame]
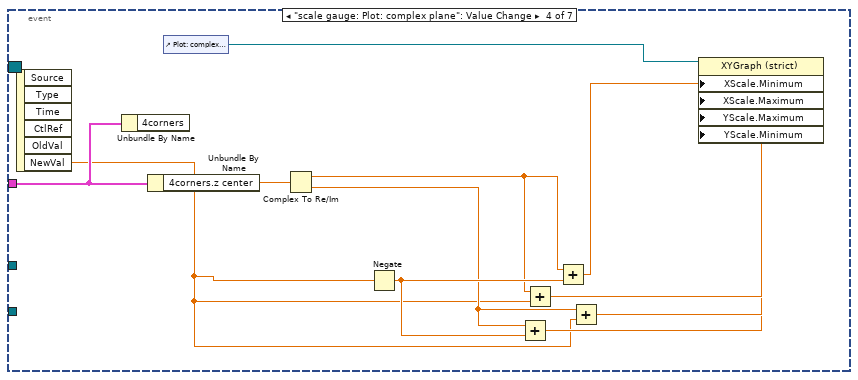
[diagram p7: hidden frame]
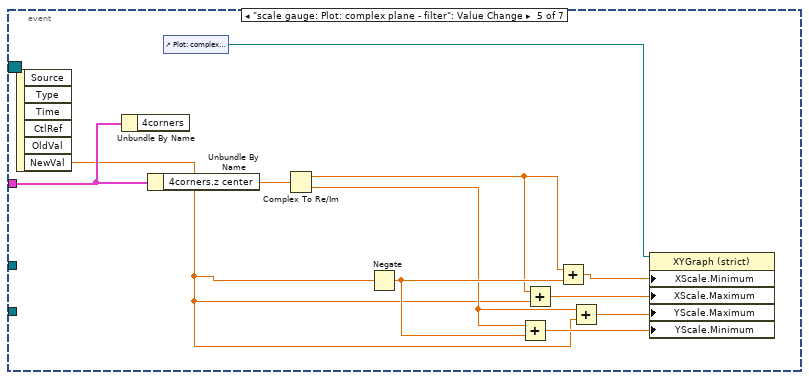
[diagram p8: hidden frame]
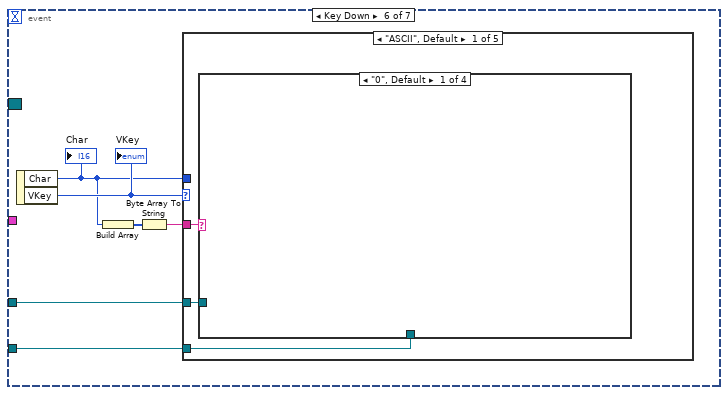
[diagram p9: hidden frame]
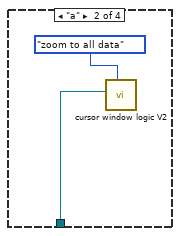
[diagram p10: hidden frame]
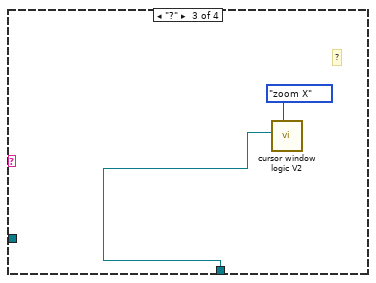
[diagram p11: hidden frame]
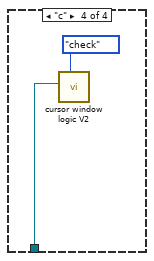
[diagram p12: hidden frame]
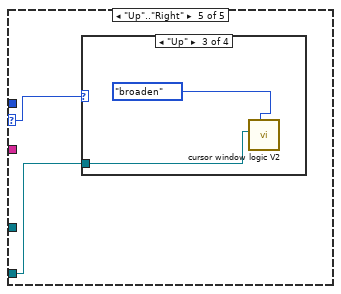
[diagram p16: hidden frame]
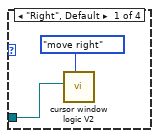
[diagram p17: hidden frame]
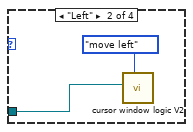
[diagram p18: hidden frame]
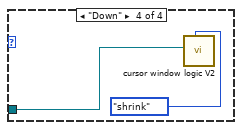
[diagram p19: hidden frame]
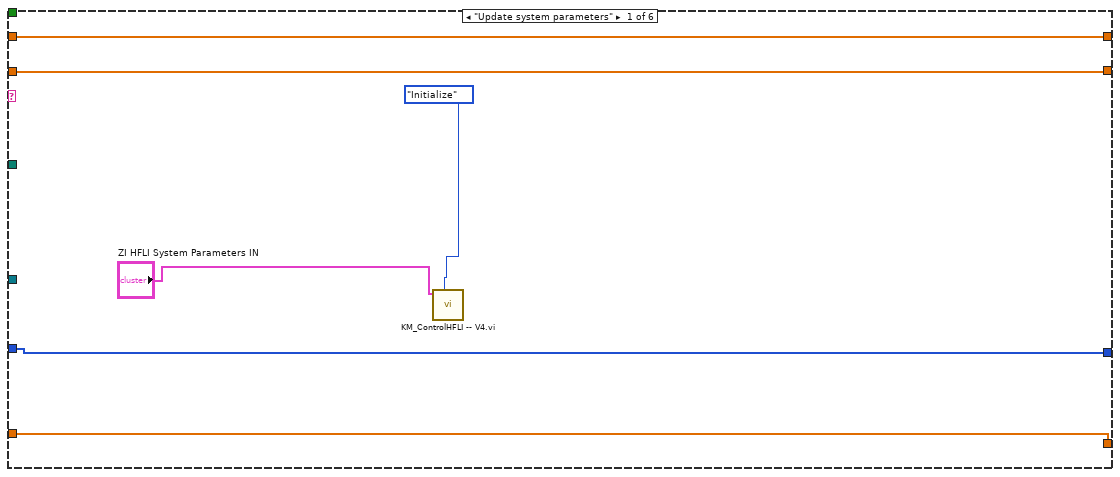
[diagram p20: hidden frame]
diagram:
  w28 = "action"  # user action
  w30 = "action"  # calculate
  (unwired) FALSE
  # "some init staff"
  n1 = control-ref of="Plot: All"() -> (w7:refnum<vi>)
  n2 = Create User Event(user event datatype=w30) -> (user event=w16:refnum<user-event>)  [unwired: 1 in, 1 out]
  n3 = Build Array(0, 1, 2) -> (w15:i32[])
  n4 = control-ref of="Plot: complex plane - filter"() -> (w25:refnum<vi>)
  n5 = control-ref of="Plot: dz/domega"() -> (w24:refnum<vi>)
  n6 = control-ref of="Plot: fragment - filter"() -> (w23:refnum<vi>)
  n7 = control-ref of="Plot: win omega"() -> (w22:refnum<vi>)
  n8 = control-ref of="Plot: phase"() -> (w21:refnum<vi>)
  n9 = control-ref of="Plot: phase around center"() -> (w19:refnum<vi>)
  n10 = control-ref of="Plot: complex plane"() -> (w18:refnum<vi>)
  n11 = control-ref of="Plot: fragment"() -> (w17:refnum<vi>)
  n12 = Bundle By Name(cluster=T3 {"left"=0.0, "right "=0.0, "center"=0.0, "window"=0.0, "cursors"=[], "relative"=0, "absolute"=0, "fixed vertical offset"=0.0, "vertical offset"=0.0, "skew"=0.0, "default window frac"=0.0, "kind"=enum."symmetric", "skew.left"=0.0, "skew.right"=0.0, "Plot ref"=refnum, "wing order"=enum."forw"} ("cursor bracket: All, data window"), "Plot ref"=w7, "cursors"=w15, "fixed vertical offset"=0.0, "default window frac"=0.3 ("fixed vertical offset"), "kind"=enum16{"symmetric", "skewed", "fancy"}."symmetric") -> (w6:T3)
  n13 = Bundle By Name(cluster=T13 {"Plot: complex plane - filter"=refnum, "Plot: dz/domega"=refnum, "Plot: fragment filter"=refnum, "Plot: win omega"=refnum, "Plot: phase"=refnum, "Plot: phase around center"=refnum, "Plot: complex plane"=refnum, "Plot: fragment"=refnum} ("plots: filter related"), "Plot: complex plane - filter"=w25, "Plot: dz/domega"=w24, "Plot: fragment filter"=w23, "Plot: win omega"=w22, "Plot: phase"=w21, "Plot: phase around center"=w19, "Plot: complex plane"=w18, "Plot: fragment"=w17) -> (w20:T13)
  n14 = control-ref of="cursor bracket: All, data window"() -> (w5:refnum<vi>)
  n15 = call "cursor window logic V2.vi"("cursor window action"=cursor_window_action."init", "cursor window in"=w5, "cursor window init"=w6) -> ("cursor window out"=w3:refnum<vi>)  [unwired: 7 in, 1 out]
  n16 = register-events(w16) -> (reference out=w31:refnum<event-registration>)  [unwired: 2 in, 1 out]
  n17 = call "cursor window logic V2.vi"("cursor window action"=cursor_window_action."check", "cursor window in"=w3) -> ("cursor window out"=w1:refnum<vi>)  [unwired: 8 in, 1 out]
  n18 = while {
    tunnel: w31 -> [w40]
    tunnel: w16 -> [w38]
    tunnel: w20 -> [w34]
    tunnel: w1 -> [w32]
    i -> [w35]
    stop <- FALSE stop-if-true
    n19 = Equal To 0?(x=w35) -> (x = 0?=w33:bool)
    n20 = event shown="[0] <calculate>: User Event" {
      selector: w40 -> [_ _]
      dyn-events: _ -> [_ _]
      timeout: 1 -> [_ _]
      tunnel: w38 -> [w48 _]
      tunnel: w34 -> [w45 _]
      tunnel: w33 -> [w44 _]
      tunnel: w32 -> [w43 _]
      event User Event {
        # "all z"
        # "all omega"
        n21 = event-data() -> ("calculate"=w49:string)  [unwired: 1 in]
        n22 = local read "pm lorentzian"() -> (w41:T6)
        n23 = Unbundle By Name(w41) -> ("omega(0)"=w42:dbl)
        n24 = for {
          N: 1 -> [_]
          tunnel: w49 -> [w65]
          tunnel: w48 -> [w64]
          shift-right: [w58] -> _
          shift-left: _ -> [w63]
          shift-right: [w57] -> _
          shift-left: _ -> [w62]
          tunnel: "Save frequency scan" -> [w61]
          tunnel: w45 -> [w60]
          tunnel: w44 -> [w59]
          tunnel: w43 -> [w56]
          tunnel: w42 -> [w55]
          tunnel: w41 -> [w54]
          shift-right: [w52] -> _
          shift-left: _ -> [w53]
          shift-right: [w51] -> _
          shift-left: _ -> [w50]
          n25 = case shown="\"Update range\"" w65 {
            tunnel: w64 -> [_ w80 _ _ _ _]
            tunnel: w63 -> [w71 _ w101 w111 w154 w164]
            tunnel: w62 -> [w70 _ w100 w110 w153 w163]
            tunnel: w61 -> [_ _ _ w106 _ _]
            tunnel: w60 -> [_ _ _ _ w155 _]
            tunnel: w59 -> [_ _ _ _ _ _]
            tunnel: [w71 w78 w101 w111 w154 w164] -> w58
            tunnel: [w70 w81 w100 w110 w153 w163] -> w57
            tunnel: w56 -> [_ _ _ w107 w150 _]
            tunnel: w55 -> [_ _ w99 _ _ _]
            tunnel: w54 -> [_ _ _ w102 _ _]
            tunnel: w53 -> [w67 w72 w97 w104 w147 w162]
            tunnel: [w67 w72 w94 w104 w147 w162] -> w52
            tunnel: [w66 w74 w96 w103 w146 w161] -> w51
            tunnel: w50 -> [w66 w74 w98 w103 w146 w161]
            frame "Update system parameters" {
              n26 = call "KM_ControlHFLI -- V4.vi.vi"("Control HFLI command"=KM_ControlHFLIcommand."Initialize", "ZI HFLI System Parameters IN"="ZI HFLI System Parameters IN") -> ()  [unwired: 4 in, 3 out]
            }
            frame "New data arrives" {
              n27 = local read "Voltage out"() -> (w81:cdb[])
              n28 = local read "Freq out"() -> (w78:dbl[])
              n29 = Complex To Re/Im(x + iy=w81) -> (x=w84:dbl[], y=w83:dbl[])
              n30 = Bundle("Freq out"=w78, w84) -> (w85:cluster{"Freq out":dbl[], dbl[]})  [unwired: 1 in]
              n31 = Bundle("Freq out"=w78, w83) -> (w82:cluster{"Freq out":dbl[], dbl[]})  [unwired: 1 in]
              n32 = Build Array(w85, w82) -> (→"Plot: All":cluster{"Freq out":dbl[], dbl[]}[])
              n33 = Generate User Event(user event=w80, event data cluster="Fit" ("event data")) -> (user event out=w76:refnum<user-event>)  [unwired: 2 in, 1 out]
              n34 = case shown="True" "Auto-update range" {
                tunnel: w76 -> [w87 w89]
                tunnel: [w87 w88] -> w75
                frame False {
                }
                frame True {
                  n35 = Generate User Event(user event=w89, event data cluster="Update range" ("event data")) -> (user event out=w88:refnum<user-event>)  [unwired: 2 in, 1 out]
                }
              }
              n36 = case shown="True" "Plot frequency shift" {
                tunnel: w75 -> [_ w91]
                frame False {
                }
                frame True {
                  n37 = Generate User Event(user event=w91, event data cluster="Plot frequency shift" ("event data")) -> ()  [unwired: 2 in, 2 out]
                }
              }
            }
            frame "Plot frequency shift" {
              n38 = Build Array (concatenate)(w98, w99) -> (w96:dbl[])
              n39 = Array Size(array=w96) -> (size(s)=w95:i32)
              n40 = Build Array (concatenate)(w97, w95) -> (w94:i32[])
              n41 = Bundle(w94, w96) -> (→"Plot: freq vs T":cluster{i32[], dbl[]})  [unwired: 1 in]
            }
            frame "Update range" {
              n42 = local read "ZI HFLI System Parameters IN"() -> (w109:T2)
              n43 = in-place {
                in-place-border: "scan monitor control" -> [w127]
                in-place-border: w107 -> [w115]
                in-place-border: w106 -> [w114]
                in-place-border: w102 -> [w113]
                in-place-border: w102 -> [w112]
                n44 = in-place-cluster #1(w109) -> ("Start (Hz)"=w117:dbl, "Stop (Hz)"=w116:dbl)
                n45 = Unbundle By Name(w113) -> ("omega(0)"=w124:dbl, "Gamma"=w119:dbl)
                n46 = Not A Number/Path/Refnum?(number/path/refnum=w119) -> (NaN/Path/Refnum?=w120:bool)
                n47 = Not A Number/Path/Refnum?(number/path/refnum=w124) -> (NaN/Path/Refnum?=w122:bool)
                n48 = Not(x=w120) -> (.not. x?=w118:bool)
                n49 = Not(x=w122) -> (.not. x?=w121:bool)
                n50 = And(x=w121, y=w118) -> (x .and. y?=w123:bool)
                n51 = case shown="True" w123 {
                  tunnel: w127 -> [_ w145]
                  tunnel: [w128 w144] -> w126
                  tunnel: w119 -> [_ w137]
                  tunnel: w124 -> [_ w139]
                  tunnel: [w129 w142] -> w125
                  tunnel: w117 -> [w129 _]
                  tunnel: w116 -> [w128 _]
                  tunnel: w115 -> [_ w140]
                  tunnel: w114 -> [_ w133]
                  tunnel: w112 -> [_ w130]
                  frame False {
                  }
                  frame True {
                    n52 = Unbundle By Name(w145) -> ("gamma-factor (fa)"=w138:dbl)
                    n53 = Compound Arithmetic op=MULTIPLY(w138, w137, 1.6 ("value")) -> (w135:dbl)
                    n54 = Multiply(x=w138, y=w137) -> (x*y=w143:dbl)
                    n55 = Add(x=w143, y=w139) -> (x+y=w144:dbl)
                    n56 = call <vilib>:"High Resolution Relative Seconds.vi"() -> ("relative seconds"=w131:dbl)
                    n57 = Subtract(x=w139, y=w143) -> (x-y=w142:dbl)
                    n58 = call "cursor window logic V2.vi"("cursor window action"=cursor_window_action."change window", "window"=w135, "center"=w139, "cursor window in"=w140) -> ()  [unwired: 6 in, 2 out]
                    n59 = call "KM_appendline.vi"("Time (s)"=w131, "name or relative path"="File name", "read/write control"=KM_file_--_read-write_control."append one line", "pm lorentzian"=w130, "Save frequency scan"=w133) -> ()  [unwired: 7 in]
                  }
                }
                n60 = in-place-cluster #1("Start (Hz)"=w125, "Stop (Hz)"=w126) -> (w108:T2)
              }
              n61 = local write "ZI HFLI System Parameters IN"(w108) -> ()
            }
            frame "Fit" {
              n62 = call "cursor window logic V2.vi"("cursor window action"=cursor_window_action."check", "cursor window in"=w150) -> ("cursor window out"=w152:T3)  [unwired: 8 in, 1 out]
              n63 = call "acquire cursor window data.vi"("z in"=w153, "omega in"=w154, "cursor window"=w152) -> ("z out"=w148:cdb[], "omega  out"=w149:dbl[])  [unwired: 4 in, 3 out]
              n64 = call "KM_peak -- find -- pm - V1.vi"("omega in"=w149, "z in"=w148, "parameters: complex fit"="parameters: complex fit", "plots: filter related"=w155, "plot staff ?"="plot staff", "just guess?"="use fast fit?", "subtract linear BG"=FALSE) -> ("pm lorentzian"=w156:T6)  [unwired: 10 in, 2 out]
              n65 = local write "pm lorentzian"(w156) -> ()
            }
            frame "Void", Default {
            }
          }
        }
      }
      event Timeout {
        n66 = event-data() -> ()  [unwired: 1 in, 2 out]
      }
    }
    n67 = Wait (ms)(milliseconds to wait=u32 0) -> ()  [unwired: 1 out]
  }
  n68 = while {
    shift-right: [w172] -> _
    shift-left: _ -> [w170]
    shift-right: [w171] -> _
    shift-left: _ -> [w169]
    tunnel: w16 -> [w168]
    tunnel: w1 -> [w165]
    stop <- FALSE stop-if-true
    n69 = case shown="True" "Take data" {
      tunnel: [w174 w186] -> w172
      tunnel: [w173 w185] -> w171
      tunnel: w170 -> [w174 _]
      tunnel: w169 -> [w173 _]
      tunnel: w168 -> [_ w187]
      tunnel: w165 -> [_ w183]
      frame False {
      }
      frame True {
        (unwired) KM_ControlHFLIcommand."Scan frequency" ("Control HFLI command")
        n70 = local read "ZI HFLI System Parameters IN"() -> (w184:T2)
        n71 = Unbundle By Name(w184) -> ("IP Address"=w178:string, "Number of Points"=w175:i32)
        n72 = call "cursor window logic V2.vi"("cursor window action"=cursor_window_action."check", "cursor window in"=w183) -> ("cursor window out"=w181:T3)  [unwired: 8 in, 1 out]
        n73 = Unbundle By Name(w181) -> ("center"=w180:dbl, "window"=w179:dbl)
        n74 = call "KM_get_sweep V1.vi.vi"("N"=w175, "omega0 (Hz)"=w180, "gamma (Hz)"=w179, "Address"=w178) -> ("freq out (Hz)"=w176:dbl[], "voltage out (V)"=w177:cdb[])  [unwired: 5 in, 1 out]
        n75 = flat-sequence {
          tunnel: w176 -> [w191]
          tunnel: [w191] -> w186
          tunnel: w177 -> [w190]
          tunnel: [w190] -> w185
          tunnel: w187 -> [w188]
          frame #0 {
            n76 = Generate User Event(user event=w188, event data cluster="New data arrives" ("event data")) -> ()  [unwired: 2 in, 2 out]
          }
        }
      }
    }
    "Freq out" <- w172
    "Voltage out" <- w171
  }
  n77 = Create User Event(user event datatype=w28) -> (user event=w27:refnum<user-event>)  [unwired: 1 in, 1 out]
  n78 = register-events(w27) -> (reference out=w29:refnum<event-registration>)  [unwired: 2 in, 1 out]
  n79 = while {
    tunnel: w29 -> [w197]
    tunnel: w16 -> [w195]
    tunnel: w1 -> [w194]
    stop <- FALSE stop-if-true
    n80 = local read "pm lorentzian"() -> (w193:T6)
    n81 = event shown="[6] \"Update system parameters\": Value Change" {
      selector: w197 -> [_ _ _ _ _ _ _]
      dyn-events: _ -> [_ _ _ _ _ _ _]
      timeout: _ -> [_ _ _ _ _ _ _]
      tunnel: w195 -> [_ _ w202 _ _ w231 w252]
      tunnel: [_ _ _ _ _ _ "Update system parameters"] -> _
      tunnel: w194 -> [_ w199 _ _ _ w227 _]
      tunnel: w193 -> [_ _ _ w207 w218 _ _]
      event Timeout {
        n82 = event-data() -> ()  [unwired: 1 in, 2 out]
      }
      event "Plot: All": Cursor Move {
        n83 = event-data() -> ("CursIdx"=w200:i32)  [unwired: 1 in, 8 out]
        n84 = call "cursor window logic V2.vi"("CursIdx"=w200, "cursor window action"=cursor_window_action."cursor moves", "cursor window in"=w199) -> ()  [unwired: 7 in, 2 out]
      }
      event "Plot: All": Cursor Release {
        n85 = event-data() -> ("CursIdx"=w201:i32)  [unwired: 1 in, 8 out]
        n86 = case shown="0..2" w201 {
          tunnel: w202 -> [_ w203]
          frame 3, Default {
          }
          frame 0..2 {
            w204 = "Fit"  # event data
            n87 = Generate User Event(user event=w203, event data cluster=w204) -> ()  [unwired: 2 in, 2 out]
          }
        }
      }
      event "scale gauge: Plot: complex plane": Value Change {
        n88 = event-data() -> ("NewVal"=w206:dbl)  [unwired: 1 in, 5 out]
        n89 = Unbundle By Name(w207) -> ()  [unwired: 1 out]
        n90 = Unbundle By Name(w207) -> ("4corners.z center"=w208:cdb)
        n91 = control-ref of="Plot: complex plane"() -> (w205:refnum<vi>)
        n92 = Complex To Re/Im(x + iy=w208) -> (x=w209:dbl, y=w210:dbl)
        n93 = Negate(x=w206) -> (-x=w215:dbl)
        n94 = Add(x=w210, y=w215) -> (x+y=w211:dbl)
        n95 = Add(x=w209, y=w206) -> (x+y=w213:dbl)
        n96 = Add(x=w209, y=w215) -> (x+y=w214:dbl)
        n97 = Add(x=w210, y=w206) -> (x+y=w212:dbl)
        n98 = property on="Property Node" class="XYGraph (strict)"(reference=w205, "XScale.Minimum"=w214, "XScale.Maximum"=w213, "YScale.Maximum"=w212, "YScale.Minimum"=w211) -> ()  [unwired: 1 in, 2 out]
      }
      event "scale gauge: Plot: complex plane - filter": Value Change {
        n99 = event-data() -> ("NewVal"=w217:dbl)  [unwired: 1 in, 5 out]
        n100 = Unbundle By Name(w218) -> ()  [unwired: 1 out]
        n101 = Unbundle By Name(w218) -> ("4corners.z center"=w219:cdb)
        n102 = control-ref of="Plot: complex plane - filter"() -> (w216:refnum<vi>)
        n103 = Complex To Re/Im(x + iy=w219) -> (x=w220:dbl, y=w221:dbl)
        n104 = Negate(x=w217) -> (-x=w226:dbl)
        n105 = Add(x=w221, y=w226) -> (x+y=w222:dbl)
        n106 = Add(x=w220, y=w217) -> (x+y=w224:dbl)
        n107 = Add(x=w220, y=w226) -> (x+y=w225:dbl)
        n108 = Add(x=w221, y=w217) -> (x+y=w223:dbl)
        n109 = property on="Property Node" class="XYGraph (strict)"(reference=w216, "XScale.Minimum"=w225, "XScale.Maximum"=w224, "YScale.Maximum"=w223, "YScale.Minimum"=w222) -> ()  [unwired: 1 in, 2 out]
      }
      event Key Down {
        n110 = event-data() -> ("Char"=w229:i16, "VKey"=w232:T8)  [unwired: 1 in]
        "Char" <- w229
        "VKey" <- w232
        n111 = Build Array(w229) -> (w230:i16[])
        n112 = Byte Array To String(unsigned byte array=w230) -> (string=w228:string)
        n113 = case shown="\"ASCII\", Default" w232 {
          selector: w232 -> [_ _ _ _ w242]
          tunnel: w229 -> [_ _ _ _ _]
          tunnel: w231 -> [w235 _ _ _ _]
          tunnel: w228 -> [w234 _ _ _ _]
          tunnel: w227 -> [w233 _ _ _ w243]
          frame "ASCII", Default {
            n114 = case shown="\"0\", Default" w234 {
              tunnel: w235 -> [_ _ _ _]
              tunnel: w233 -> [_ w236 w238 w240]
              frame "0", Default {
              }
              frame "a" {
                n115 = call "cursor window logic V2.vi"("cursor window action"=cursor_window_action."zoom to all data", "cursor window in"=w236) -> ()  [unwired: 8 in, 2 out]
              }
              frame "?" {
                # "?"
                n116 = call "cursor window logic V2.vi"("cursor window action"=cursor_window_action."zoom X", "cursor window in"=w238) -> ()  [unwired: 8 in, 2 out]
              }
              frame "c" {
                n117 = call "cursor window logic V2.vi"("cursor window action"=cursor_window_action."check", "cursor window in"=w240) -> ()  [unwired: 8 in, 2 out]
              }
            }
          }
          frame "Escape" {
          }
          frame "PageUp" {
          }
          frame "PageDown" {
          }
          frame "Up".."Right" {
            n118 = case shown="\"Up\"" w242 {
              tunnel: w243 -> [w244 w246 w248 w251]
              frame "Right", Default {
                n119 = call "cursor window logic V2.vi"("cursor window action"=cursor_window_action."move right", "cursor window in"=w244) -> ()  [unwired: 8 in, 2 out]
              }
              frame "Left" {
                n120 = call "cursor window logic V2.vi"("cursor window action"=cursor_window_action."move left", "cursor window in"=w246) -> ()  [unwired: 8 in, 2 out]
              }
              frame "Up" {
                n121 = call "cursor window logic V2.vi"("cursor window action"=cursor_window_action."broaden", "cursor window in"=w248) -> ()  [unwired: 8 in, 2 out]
              }
              frame "Down" {
                n122 = call "cursor window logic V2.vi"("cursor window action"=cursor_window_action."shrink", "cursor window in"=w251) -> ()  [unwired: 8 in, 2 out]
              }
            }
          }
        }
      }
      event "Update system parameters": Value Change {
        n123 = event-data() -> ()  [unwired: 1 in, 6 out]
        n124 = Generate User Event(user event=w252, event data cluster="Update system parameters" ("event data")) -> ()  [unwired: 2 in, 2 out]
      }
    }
    n125 = Wait (ms)(milliseconds to wait=u32 0) -> ()  [unwired: 1 out]
  }
